vi "CAN_CANFD_Demo.vi"(11 "Receive":string="CAN_CANFD_Demo") -> ()   [LabVIEW 2014]
uses:
  <vilib>/Utility/miscctls.llb/LVPointTypeDef.ctl
  Utilities/Typedef/Hardware_Subtype.ctl
  TSMaster_API/CAN_CANFD_Function/Typedef/TSCAN_Config_parameter.ctl
  TSMaster_API/CAN_CANFD_Function/Typedef/TSCAN_Send_parameter.ctl
  TSMaster_API/CAN_CANFD_Function/Typedef/TSCAN_CAN_CANFD_Demo_Data.ctl
  TSMaster_API/CAN_CANFD_Function/Typedef/TSCAN_CAN_CANFD_Demo_Data1.ctl
  TSMaster_API/CAN_CANFD_Function/Typedef/TLibCANFD.ctl
  TSMaster_API/CAN_CANFD_Function/Typedef/TSCAN_DBC_Ctr.ctl
  TSMaster_API/CAN_CANFD_Function/Typedef/TSCAN_CANFD_Configuration.ctl
  TSMaster_API/CAN_CANFD_Function/Typedef/TSCAN_CAN_Configuration.ctl
  TSMaster_API/CAN_CANFD_Function/Typedef/TSCAN_CANFD_Configuration_Regs.ctl
  TSMaster_API/CAN_CANFD_Function/Typedef/TSCAN_CAN_Configuration_Regs.ctl
  TSMaster_API/All_Control/Typedef/Hardware Type.ctl
  TSMaster_API/All_Control/Typedef/Blf_Log.ctl
  TSMaster_API/DataBase/Typedef/DBSignal.ctl
  TSMaster_API/DataBase/Typedef/DBMessage.ctl
  <vilib>/regexp/Match Regular Expression.xnode
  TSMaster_API/Diagnosis/Typedef/UDS Control.ctl
  TSMaster_API/Diagnosis/Typedef/UDS Cluster.ctl
panel:
  in  "Diagram shown":bool
  in  "Stop Log":bool
  in  "Start Log":bool
  in  "log":i32(listbox)
  out "program loop":i32
  in  "Config":bool
  in  "Connect":bool
  in  "Disconnect":bool
  out "Connect ?":bool
  in  "选项卡控件":enum32{"Setting", "CAN/CANFD", "DBC_Load"}(tab)
  in  "CH_Mapping":bool
  in  "TS_Mapping":bool
  in  "BLF_Log_PATH":path
  in  "Advance_Tag":enum32{"Ordinary", "Advanced"}(tab)
  in  "CAN_Config_Array":T1[](array[typedef]) {"AAppChannel" items=["CHN1", "CHN2", "CHN3", "CHN4", "CHN5", "CHN6", "CHN7", "CHN8", "CHN9", "CHN10", "CHN11", "CHN12", "CHN13", "CHN14", "CHN15", "CHN16", "CHN17", "CHN18", "CHN19", "CHN20", "CHN21", "CHN22", "CHN23", "CHN24", "CHN25", "CHN26", "CHN27", "CHN28", "CHN29", "CHN30", "CHN31", "CHN32"]; "AHwChannel" items=["CHN1", "CHN2", "CHN3", "CHN4", "CHN5", "CHN6", "CHN7", "CHN8", "CHN9", "CHN10", "CHN11", "CHN12", "CHN13", "CHN14", "CHN15", "CHN16", "CHN17", "CHN18", "CHN19", "CHN20", "CHN21", "CHN22", "CHN23", "CHN24", "CHN25", "CHN26", "CHN27", "CHN28", "CHN29", "CHN30", "CHN31", "CHN32"]; "HardwareType" items=["BUS_UNKNOWN_TYPE", "TS_TCP_DEVICE", "XL_USB_DEVICE", "TS_USB_DEVICE", "PEAK_USB_DEVICE", "KVASER_USB_DEVICE", "ZLG_USB_DEVICE", "ICS_USB_DEVICE", "TS_TC1005_DEVICE", "CANABLE_USB_DEVICE", "TS_WIRELESS_OBD", "TS_USB_DEVICE_EX", "IXXAT_USB_DEVICE", "TS_ETH_IF_DEVICE", "TS_USB_IF_DEVICE", "BUS_DEV_TYPE_COUNT"]}
  in  "CANFD_Config_Array":T4[](array[typedef]) {"Hardware Type" items=["BUS_UNKNOWN_TYPE", "TS_TCP_DEVICE", "XL_USB_DEVICE", "TS_USB_DEVICE", "PEAK_USB_DEVICE", "KVASER_USB_DEVICE", "ZLG_USB_DEVICE", "ICS_USB_DEVICE", "TS_TC1005_DEVICE", "CANABLE_USB_DEVICE", "TS_WIRELESS_OBD", "TS_USB_DEVICE_EX", "IXXAT_USB_DEVICE", "TS_ETH_IF_DEVICE", "TS_USB_IF_DEVICE", "BUS_DEV_TYPE_COUNT"]; "AHwChannel" items=["CHN1", "CHN2", "CHN3", "CHN4", "CHN5", "CHN6", "CHN7", "CHN8", "CHN9", "CHN10", "CHN11", "CHN12", "CHN13", "CHN14", "CHN15", "CHN16", "CHN17", "CHN18", "CHN19", "CHN20", "CHN21", "CHN22", "CHN23", "CHN24", "CHN25", "CHN26", "CHN27", "CHN28", "CHN29", "CHN30", "CHN31", "CHN32"]; "AAppChannel" items=["CHN1", "CHN2", "CHN3", "CHN4", "CHN5", "CHN6", "CHN7", "CHN8", "CHN9", "CHN10", "CHN11", "CHN12", "CHN13", "CHN14", "CHN15", "CHN16", "CHN17", "CHN18", "CHN19", "CHN20", "CHN21", "CHN22", "CHN23", "CHN24", "CHN25", "CHN26", "CHN27", "CHN28", "CHN29", "CHN30", "CHN31", "CHN32"]; "AControllerType" items=["lfdtCAN", "lfdtISOFDCAN", "lfdtNonISOFDFDCAN"]; "AControllerMode" items=["lfdmNormal", "lfdmACKOff", "lfdmRestricted"]}
  in  "CANFD_Config_Regs_Array":T5[](array[typedef]) {"CANFD Configuration"."Hardware Type" items=["BUS_UNKNOWN_TYPE", "TS_TCP_DEVICE", "XL_USB_DEVICE", "TS_USB_DEVICE", "PEAK_USB_DEVICE", "KVASER_USB_DEVICE", "ZLG_USB_DEVICE", "ICS_USB_DEVICE", "TS_TC1005_DEVICE", "CANABLE_USB_DEVICE", "TS_WIRELESS_OBD", "TS_USB_DEVICE_EX", "IXXAT_USB_DEVICE", "TS_ETH_IF_DEVICE", "TS_USB_IF_DEVICE", "BUS_DEV_TYPE_COUNT"]; "CANFD Configuration"."AHwChannel" items=["CHN1", "CHN2", "CHN3", "CHN4", "CHN5", "CHN6", "CHN7", "CHN8", "CHN9", "CHN10", "CHN11", "CHN12", "CHN13", "CHN14", "CHN15", "CHN16", "CHN17", "CHN18", "CHN19", "CHN20", "CHN21", "CHN22", "CHN23", "CHN24", "CHN25", "CHN26", "CHN27", "CHN28", "CHN29", "CHN30", "CHN31", "CHN32"]; "CANFD Configuration"."AAppChannel" items=["CHN1", "CHN2", "CHN3", "CHN4", "CHN5", "CHN6", "CHN7", "CHN8", "CHN9", "CHN10", "CHN11", "CHN12", "CHN13", "CHN14", "CHN15", "CHN16", "CHN17", "CHN18", "CHN19", "CHN20", "CHN21", "CHN22", "CHN23", "CHN24", "CHN25", "CHN26", "CHN27", "CHN28", "CHN29", "CHN30", "CHN31", "CHN32"]; "CANFD Configuration"."AControllerType" items=["lfdtCAN", "lfdtISOFDCAN", "lfdtNonISOFDFDCAN"]; "CANFD Configuration"."AControllerMode" items=["lfdmNormal", "lfdmACKOff", "lfdmRestricted"]}
  in  "CAN_Config_Regs_Array":T6[](array[typedef]) {"CAN configuration"."AAppChannel" items=["CHN1", "CHN2", "CHN3", "CHN4", "CHN5", "CHN6", "CHN7", "CHN8", "CHN9", "CHN10", "CHN11", "CHN12", "CHN13", "CHN14", "CHN15", "CHN16", "CHN17", "CHN18", "CHN19", "CHN20", "CHN21", "CHN22", "CHN23", "CHN24", "CHN25", "CHN26", "CHN27", "CHN28", "CHN29", "CHN30", "CHN31", "CHN32"]; "CAN configuration"."AHwChannel" items=["CHN1", "CHN2", "CHN3", "CHN4", "CHN5", "CHN6", "CHN7", "CHN8", "CHN9", "CHN10", "CHN11", "CHN12", "CHN13", "CHN14", "CHN15", "CHN16", "CHN17", "CHN18", "CHN19", "CHN20", "CHN21", "CHN22", "CHN23", "CHN24", "CHN25", "CHN26", "CHN27", "CHN28", "CHN29", "CHN30", "CHN31", "CHN32"]; "CAN configuration"."HardwareType" items=["BUS_UNKNOWN_TYPE", "TS_TCP_DEVICE", "XL_USB_DEVICE", "TS_USB_DEVICE", "PEAK_USB_DEVICE", "KVASER_USB_DEVICE", "ZLG_USB_DEVICE", "ICS_USB_DEVICE", "TS_TC1005_DEVICE", "CANABLE_USB_DEVICE", "TS_WIRELESS_OBD", "TS_USB_DEVICE_EX", "IXXAT_USB_DEVICE", "TS_ETH_IF_DEVICE", "TS_USB_IF_DEVICE", "BUS_DEV_TYPE_COUNT"]}
  in  "DLL_PATH":path
  in  "Bus_Type":u16(ring) items=["CAN", "CANFD"]
  in  "Channels used":u16(ring)=1 items=["1 Channel"=1, "2 Channels"=2, "3 Channels"=3, "4 Channels"=4, "5 Channels"=5, "6 Channels"=6, "7 Channels"=7, "8 Channels"=8, "9 Channels"=9, "10 Channels"=10, "11 Channels"=11, "12 Channels"=12, "13 Channels"=13, "14 Channels"=14, "15 Channels"=15, "16 Channels"=16]
  in  "Sampling point":bool
  in  "Export":bool
  in  "Import":bool
  in  "REC_Channel":i32(ring) items=["CHN1", "CHN2", "CHN3", "CHN4", "CHN5", "CHN6", "CHN7", "CHN8", "CHN9", "CHN10", "CHN11", "CHN12", "CHN13", "CHN14", "CHN15", "CHN16", "CHN17", "CHN18", "CHN19", "CHN20", "CHN21", "CHN22", "CHN23", "CHN24", "CHN25", "CHN26", "CHN27", "CHN28", "CHN29", "CHN30", "CHN31", "CHN32"]
  in  "DIS_REC":bool
  in  "Pause":bool
  in  "Read message type":u16(ring)=1 items=["Only read received messages", "Receive&send messages"]
  out "Receive Status":bool
  in  "Clear":bool
  in  "BRS":enum16{"Close", "Open"}(ring)
  in  "FD Frame":u8(ring) items=["Ordinary CAN Data", "FD CAN Data"]
  in  "Frame Type":u8(ring) items=["Data Frame", "Remote Frame", ""]
  in  "Frame Format":u8(ring) items=["Standard Frame", "Extended Frame"]
  in  "ID":i32 format="%x"
  in  "Data Length":i32(ring)=15 items=["0", "1", "2", "3", "4", "5", "6", "7", "8", "12", "16", "20", "24", "32", "48", "64"]
  in  "SendData":u8[](array[numeric])=[0, 0, 0, 0, 0, 0, 0, 0, 0, 0, 0, 0, 0, 0, 0, 0, 0, 0, 0, 0, 0, 0, 0, 0, 0, 0, 0, 0, 0, 0, 0, 0, 0, 0, 0, 0, 0, 0, 0, 0, 0, 0, 0, 0, 0, 0, 0, 0, 0, 0, 0, 0, 0, 0, 0, 0, 0, 0, 0, 0, 0, 0, 0, 0, 0, 0, 0, 0, 0, 0, 0, 0, 0, 0, 0] format="%x"
  in  "Data":i32(listbox)=-1
  in  "Send_Tag":T7(tab)
  out "ms":u32
  out "send successful?":bool
  in  "Sending":bool
  in  "Cycle":bool=TRUE
  in  "Channel":i32(ring) items=["CHN1", "CHN2", "CHN3", "CHN4", "CHN5", "CHN6", "CHN7", "CHN8", "CHN9", "CHN10", "CHN11", "CHN12", "CHN13", "CHN14", "CHN15", "CHN16", "CHN17", "CHN18", "CHN19", "CHN20", "CHN21", "CHN22", "CHN23", "CHN24", "CHN25", "CHN26", "CHN27", "CHN28", "CHN29", "CHN30", "CHN31", "CHN32"]
  in  "async&sync":u16(ring) items=["async", "sync"]
  in  "Timeout":u16
  in  "Periodic_Send":bool
  in  "Filtering":bool
  in  "DBC_Send":bool
  in  "AsynCall":bool
  in  "UDS":bool
  out "BufferCount":i32
  out "ok?":bool
  out "State":dbl
  out "Stste?":bool
  in  "AIdxStat":i32(ring) items=["cbsBusLoad", "cbsPeakLoad", "cbsFpsStdData", "cbsAllStdData", "cbsFpsExtData", "cbsAllExtData", "cbsFpsStdRemote", "cbsAllStdRemote", "cbsFpsExtRemote", "cbsAllExtRemote", "cbsFpsErrorFrame", "cbsAllErrorFrame"]
  in  "Fold Data":bool
  out "Laod BDC Successful?":bool
  in  "DBC Tab":enum32{"Message", "Signal"}(tab) caption="Tab Control 2"
  in  "Message Table":string[][](table)=[["Name", ""], ["Type", ""], ["Data Length", ""], ["Identifier", ""], ["Baud rate switching flag", ""], ["Cycle (milliseconds)", ""], ["Annotation", ""]]
  in  "Signal Table":string[][](table)=[["Name", ""], ["Length", ""], ["Endian", ""], ["DataType", ""], ["Minimum", ""], ["Maximum", ""], ["Unit", ""], ["Factor", ""], ["Offset", ""], ["InitiaValue", ""], ["Annotation", ""]]
  in  "GetCount_DBC":bool
  in  "Unload_DBC":bool
  in  "Load_DBC":bool
  in  "Tree control":string(tree)
  in  "DBC loading channel":i32(ring) items=["CHN1", "CHN2", "CHN3", "CHN4", "CHN5", "CHN6", "CHN7", "CHN8", "CHN9", "CHN10", "CHN11", "CHN12", "CHN13", "CHN14", "CHN15", "CHN16", "CHN17", "CHN18", "CHN19", "CHN20", "CHN21", "CHN22", "CHN23", "CHN24", "CHN25", "CHN26", "CHN27", "CHN28", "CHN29", "CHN30", "CHN31", "CHN32"]
  in  "DBC Path":path
  in  "STOP":bool
  # "CAN/CANFD Demo"
  # "Please click the 'Config' button first,Don't click \"Connect\""
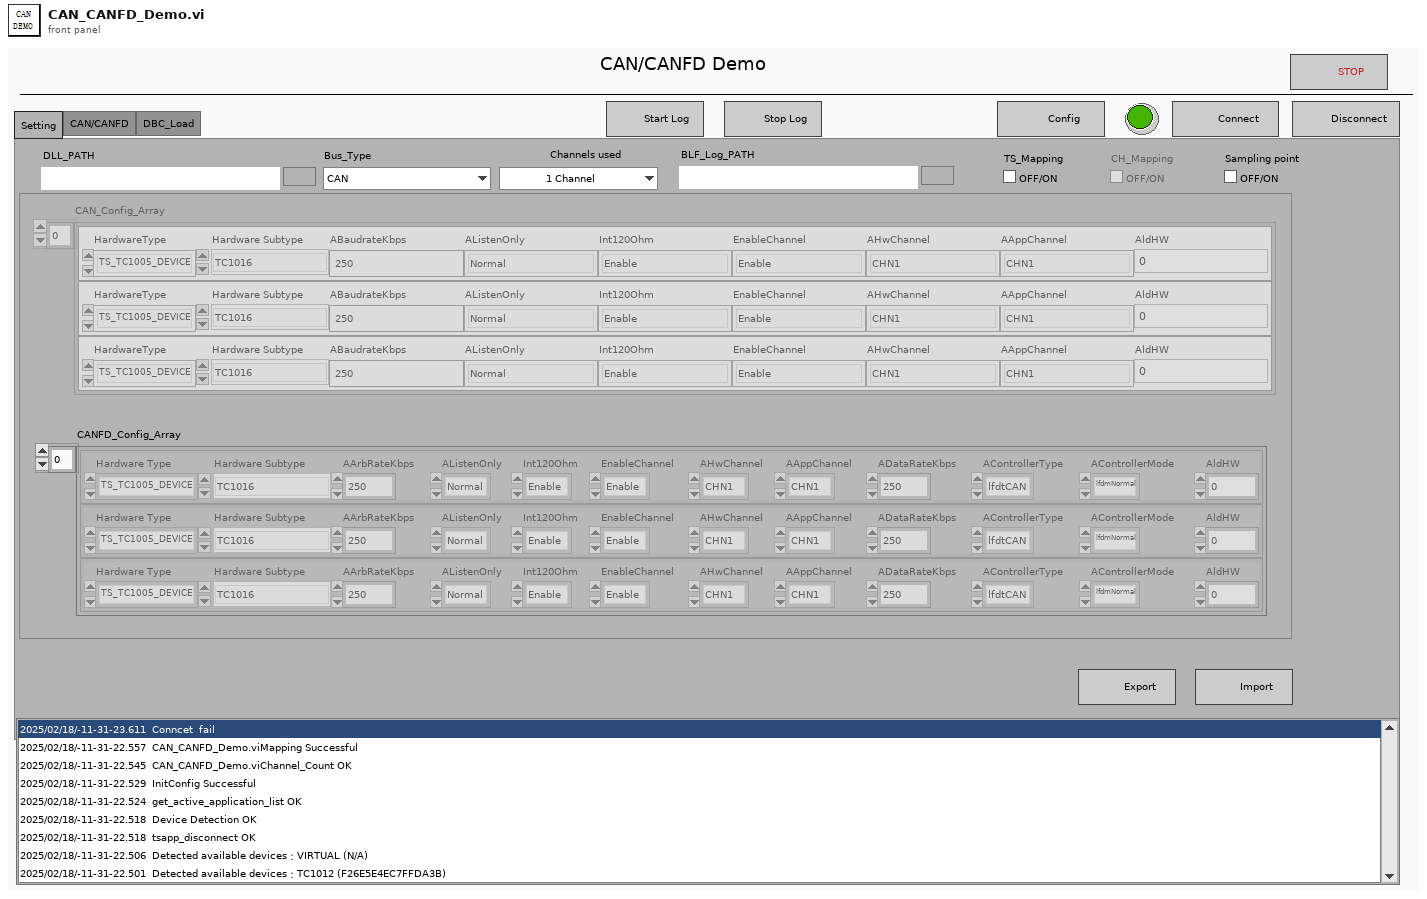
[diagram p1: front panel]
types:
  T1 = typedef "TSCAN_CAN_Configuration.ctl" = cluster{"HardwareType":T2, "Hardware Subtype":T3, "ABaudrateKbps":sgl, "AListenOnly":enum16{"Normal", "ListenOnly"}, "Int120Ohm":enum16{"Disable", "Enable"}, "EnableChannel":enum16{"Disable", "Enable"}, "AHwChannel":i32, "AAppChannel":i32, "AldHW":i32}
  T2 = typedef "Hardware Type.ctl" = i32
  T3 = typedef "Hardware_Subtype.ctl" = enum16{"TS_UNKNOWN_DEVICE", "TSCAN_PRO", "TSCAN_Lite1", "TC1001", "TL1001", "TC1011", "TM5011", "TC1002", "TC1014", "TSCANFD2517", "TC1026", "TC1016", "TC1012", "TC1013", "TLog1002", "TC1034", "TC1018", "GW2116", "TC2115", "MP1013", "TC1113", "TC1114", "TP1013", "TC1017", "TP1018", "TF10XX", "TL1004_FD_4_LIN_2", "TE1051", "TP1051", "TP1034", "TTS9015", "TP1026", "TTS1026", "TTS1034", "TTS1018", "TL1011", "TTS1015_LiAuto", "TTS1013_LiAuto", "TTS1016Pro", "TC1054Pro", "TC1054", "TLog1038", "TO1013", "TC1034Pro", "TC1018Pro", "TC1038Pro", "TS_DEV_END"}
  T4 = typedef "TSCAN_CANFD_Configuration.ctl" = cluster{"Hardware Type":T2, "Hardware Subtype":T3, "AArbRateKbps":sgl, "AListenOnly":enum16{"Normal", "ListenOnly"}, "Int120Ohm":enum16{"Disable", "Enable"}, "EnableChannel":enum16{"Disable", "Enable"}, "AHwChannel":i32, "AAppChannel":i32, "ADataRateKbps":sgl, "AControllerType":i32, "AControllerMode":i32, "AldHW":i32}
  T5 = typedef "TSCAN_CANFD_Configuration_Regs.ctl" = cluster{"CANFD Configuration":T4, "CANFD_Sampling point":cluster{"AArbSEG1":i32, "AArbSEG2":i32, "AArbPrescaler":i32, "AArbSJW":i32, "ADataSEG1":i32, "ADataSEG2":i32, "ADataPrescaler":i32, "ADataSJW":i32}}
  T6 = typedef "TSCAN_CAN_Configuration_Regs.ctl" = cluster{"CAN_Sampling point":cluster{"ASEG1":i32, "ASEG2":i32, "APrescaler":i32, "ASJW":i32}, "CAN configuration":T1}
  T7 = enum32{"Single step", "Periodic", "Filter_Pass", "DBC", "UDS"}
  T8 = enum8{"Enabled", "Disabled", "Disabled and Grayed Out"}
  T9 = typedef "LVPointTypeDef.ctl" = cluster{"Horizontal":i16, "Vertical":i16}
  T10 = typedef "TSCAN_CAN_CANFD_Demo_Data1.ctl" = cluster{"Communication message":cluster{"Sender":string, "receiver":string, "message":string, "data":variant}, "Data":T11, "CAN_Buffer":cluster{"FIdxChn":u8, "FProperties":u8, "FDLC":u8, "FReserved":u8, "FIdentifier":i32, "FTimeUS":u64, "FData":cluster{"Data0":u8, "Data1":u8, "Data2":u8, "Data3":u8, "Data4":u8, "Data5":u8, "Data6":u8, "Data7":u8}}[], "CANFD_Buffer":cluster{"FIdxChn":u8, "FProperties":u8, "FDLC":u8, "FReserved":u8, "FIdentifier":i32, "FTimeUS":u64, "FDatas":cluster{"Initialize array[0]":u8, "Initialize array[1]":u8, "Initialize array[2]":u8, "Initialize array[3]":u8, "Initialize array[4]":u8, "Initialize array[5]":u8, "Initialize array[6]":u8, "Initialize array[7]":u8, "Initialize array[8]":u8, "Initialize array[9]":u8, "Initialize array[10]":u8, "Initialize array[11]":u8, "Initialize array[12]":u8, "Initialize array[13]":u8, "Initialize array[14]":u8, "Initialize array[15]":u8, "Initialize array[16]":u8, "Initialize array[17]":u8, "Initialize array[18]":u8, "Initialize array[19]":u8, "Initialize array[20]":u8, "Initialize array[21]":u8, "Initialize array[22]":u8, "Initialize array[23]":u8, "Initialize array[24]":u8, "Initialize array[25]":u8, "Initialize array[26]":u8, "Initialize array[27]":u8, "Initialize array[28]":u8, "Initialize array[29]":u8, "Initialize array[30]":u8, "Initialize array[31]":u8, "Initialize array[32]":u8, "Initialize array[33]":u8, "Initialize array[34]":u8, "Initialize array[35]":u8, "Initialize array[36]":u8, "Initialize array[37]":u8, "Initialize array[38]":u8, "Initialize array[39]":u8, "Initialize array[40]":u8, "Initialize array[41]":u8, "Initialize array[42]":u8, "Initialize array[43]":u8, "Initialize array[44]":u8, "Initialize array[45]":u8, "Initialize array[46]":u8, "Initialize array[47]":u8, "Initialize array[48]":u8, "Initialize array[49]":u8, "Initialize array[50]":u8, "Initialize array[51]":u8, "Initialize array[52]":u8, "Initialize array[53]":u8, "Initialize array[54]":u8, "Initialize array[55]":u8, "Initialize array[56]":u8, "Initialize array[57]":u8, "Initialize array[58]":u8, "Initialize array[59]":u8, "Initialize array[60]":u8, "Initialize array[61]":u8, "Initialize array[62]":u8, "Initialize array[63]":u8}}[], "error in":errorcluster, "CAN_Period_Datas":cluster{"FIdxChn":u8, "FProperties":u8, "FDLC":u8, "FReserved":u8, "FIdentifier":i32, "FTimeUS":u64, "FData":cluster{"Data0":u8, "Data1":u8, "Data2":u8, "Data3":u8, "Data4":u8, "Data5":u8, "Data6":u8, "Data7":u8}}[], "CANFD_period_Datas":cluster{"FIdxChn":u8, "FProperties":u8, "FDLC":u8, "FReserved":u8, "FIdentifier":i32, "FTimeUS":u64, "FDatas":cluster{"Initialize array[0]":u8, "Initialize array[1]":u8, "Initialize array[2]":u8, "Initialize array[3]":u8, "Initialize array[4]":u8, "Initialize array[5]":u8, "Initialize array[6]":u8, "Initialize array[7]":u8, "Initialize array[8]":u8, "Initialize array[9]":u8, "Initialize array[10]":u8, "Initialize array[11]":u8, "Initialize array[12]":u8, "Initialize array[13]":u8, "Initialize array[14]":u8, "Initialize array[15]":u8, "Initialize array[16]":u8, "Initialize array[17]":u8, "Initialize array[18]":u8, "Initialize array[19]":u8, "Initialize array[20]":u8, "Initialize array[21]":u8, "Initialize array[22]":u8, "Initialize array[23]":u8, "Initialize array[24]":u8, "Initialize array[25]":u8, "Initialize array[26]":u8, "Initialize array[27]":u8, "Initialize array[28]":u8, "Initialize array[29]":u8, "Initialize array[30]":u8, "Initialize array[31]":u8, "Initialize array[32]":u8, "Initialize array[33]":u8, "Initialize array[34]":u8, "Initialize array[35]":u8, "Initialize array[36]":u8, "Initialize array[37]":u8, "Initialize array[38]":u8, "Initialize array[39]":u8, "Initialize array[40]":u8, "Initialize array[41]":u8, "Initialize array[42]":u8, "Initialize array[43]":u8, "Initialize array[44]":u8, "Initialize array[45]":u8, "Initialize array[46]":u8, "Initialize array[47]":u8, "Initialize array[48]":u8, "Initialize array[49]":u8, "Initialize array[50]":u8, "Initialize array[51]":u8, "Initialize array[52]":u8, "Initialize array[53]":u8, "Initialize array[54]":u8, "Initialize array[55]":u8, "Initialize array[56]":u8, "Initialize array[57]":u8, "Initialize array[58]":u8, "Initialize array[59]":u8, "Initialize array[60]":u8, "Initialize array[61]":u8, "Initialize array[62]":u8, "Initialize array[63]":u8}}[], "CAN_Filtering_Datas":cluster{"FIdxChn":u8, "FProperties":u8, "FDLC":u8, "FReserved":u8, "FIdentifier":i32, "FTimeUS":u64, "FData":cluster{"Data0":u8, "Data1":u8, "Data2":u8, "Data3":u8, "Data4":u8, "Data5":u8, "Data6":u8, "Data7":u8}}[], "CANFD_Filtering_Datas":cluster{"FIdxChn":u8, "FProperties":u8, "FDLC":u8, "FReserved":u8, "FIdentifier":i32, "FTimeUS":u64, "FDatas":cluster{"Initialize array[0]":u8, "Initialize array[1]":u8, "Initialize array[2]":u8, "Initialize array[3]":u8, "Initialize array[4]":u8, "Initialize array[5]":u8, "Initialize array[6]":u8, "Initialize array[7]":u8, "Initialize array[8]":u8, "Initialize array[9]":u8, "Initialize array[10]":u8, "Initialize array[11]":u8, "Initialize array[12]":u8, "Initialize array[13]":u8, "Initialize array[14]":u8, "Initialize array[15]":u8, "Initialize array[16]":u8, "Initialize array[17]":u8, "Initialize array[18]":u8, "Initialize array[19]":u8, "Initialize array[20]":u8, "Initialize array[21]":u8, "Initialize array[22]":u8, "Initialize array[23]":u8, "Initialize array[24]":u8, "Initialize array[25]":u8, "Initialize array[26]":u8, "Initialize array[27]":u8, "Initialize array[28]":u8, "Initialize array[29]":u8, "Initialize array[30]":u8, "Initialize array[31]":u8, "Initialize array[32]":u8, "Initialize array[33]":u8, "Initialize array[34]":u8, "Initialize array[35]":u8, "Initialize array[36]":u8, "Initialize array[37]":u8, "Initialize array[38]":u8, "Initialize array[39]":u8, "Initialize array[40]":u8, "Initialize array[41]":u8, "Initialize array[42]":u8, "Initialize array[43]":u8, "Initialize array[44]":u8, "Initialize array[45]":u8, "Initialize array[46]":u8, "Initialize array[47]":u8, "Initialize array[48]":u8, "Initialize array[49]":u8, "Initialize array[50]":u8, "Initialize array[51]":u8, "Initialize array[52]":u8, "Initialize array[53]":u8, "Initialize array[54]":u8, "Initialize array[55]":u8, "Initialize array[56]":u8, "Initialize array[57]":u8, "Initialize array[58]":u8, "Initialize array[59]":u8, "Initialize array[60]":u8, "Initialize array[61]":u8, "Initialize array[62]":u8, "Initialize array[63]":u8}}[], "AsynCall?":bool}
  T11 = typedef "TSCAN_CAN_CANFD_Demo_Data.ctl" = cluster{"Config_parameter":T12, "Send_parameter":T13, "DBC_Ctr":T14, "CAN_Config_Array":T1[], "CANFD_Config_Array":T4[], "CAN_Config_Regs_Array":T6[], "CANFD_Config_Regs_Array":T5[], "Blf_Log":T17, "UDS":T18}
  T12 = typedef "TSCAN_Config_parameter.ctl" = cluster{"Bus_Type":u16, "Channel":i32, "Channels used":u16, "DLL_PATH":path, "Read message type":u16, "REC_Channel":i32}
  T13 = typedef "TSCAN_Send_parameter.ctl" = cluster{"SendData":u8[], "Data Length":i32, "ID":i32, "Frame Format":u8, "Frame Type":u8, "BRS":enum16{"Close", "Open"}, "FD Frame":u8, "async&sync":enum16{"async", "sync"}, "Timeout":u16}
  T14 = typedef "TSCAN_DBC_Ctr.ctl" = cluster{"DBC Path":path, "DBC loading channel":i32, "DatabaseId":u32, "DBMessages":T15[], "DBSignals":cluster{"MessageName":string, "SignalList":T16[]}[]}
  T15 = typedef "DBMessage.ctl" = cluster{"Type":u16, "DLC":i32, "ID":i32, "CycleTime":dbl, "Name":string, "Comment":string, "TX_Node_Index":i32, "Owned_Signal_List_Count ":i32, "Owned_Signal_List_Signal_Index":i32, "BRS":i32}
  T16 = typedef "DBSignal.ctl" = cluster{"ID":i32, "Value_Type":i32, "Is_Motorola":i32, "ValTab_Index":i32, "Mux_Type":i32, "Mux_Value":dbl, "Layout_Start":i32, "Length":i32, "Factor":dbl, "Offset":dbl, "InitValue":dbl, "Min":dbl, "Max":dbl, "Name":string, "Unit":string, "Comment":string, "Message_Index":i32, "Message_Type":i32}
  T17 = typedef "Blf_Log.ctl" = cluster{"Blf_Log_PATH":path}
  T18 = typedef "UDS Cluster.ctl" = cluster{"UDS Control":T19, "DiagModuleIndex":i32}
  T19 = typedef "UDS Control.ctl" = cluster{"UDS Channel Index":u32, "Request ID":u32, "Response ID":u32, "Request ID (Func)":u32, "Session Mode":u8, "Reset Mode":u8, "DTC Mask":u8, "GropOfDTC":u32, "Seed Level":i32, "Seed":u8[], "Key Level":i32, "Key":u8[], "Read Identifier":u16, "UDS Read Data":u8[], "ASCII Data":string, "Write Identifier":u16, "UDS Wrtie Data":u8[], "IO Control Identifier":u16, "UDS IOControl Data":u8[], "IO Control Mode":u8, "UDS IOControl Read Data":u8[], "Routine Control Identifier":u16, "UDS RoutineControl Data":u8[], "UDS RoutineControl Read Data":u8[], "Routine Control Mode":u8, "SupportFDCAN":bool, "time config":cluster{"p2_timeout":i32, "p2_extended":i32, "s3_servertime":i32, "s3_clienttime":i32}, "ServiceLayer":cluster{"FilledByte":u8, "STMin":i32, "BlockSize":i32, "FCDelay":i32, "MaxLength":i32}, "Request":u8[], "Respond":u8[]}
  T20 = cluster{"Sender":string, "receiver":string, "message":string, "data":variant}
  T21 = cluster{"FIdxChn":u8, "FProperties":u8, "FDLC":u8, "FReserved":u8, "FIdentifier":i32, "FTimeUS":u64, "FData":cluster{"Data0":u8, "Data1":u8, "Data2":u8, "Data3":u8, "Data4":u8, "Data5":u8, "Data6":u8, "Data7":u8}}[]
  T22 = cluster{"FIdxChn":u8, "FProperties":u8, "FDLC":u8, "FReserved":u8, "FIdentifier":i32, "FTimeUS":u64, "FDatas":cluster{"Initialize array[0]":u8, "Initialize array[1]":u8, "Initialize array[2]":u8, "Initialize array[3]":u8, "Initialize array[4]":u8, "Initialize array[5]":u8, "Initialize array[6]":u8, "Initialize array[7]":u8, "Initialize array[8]":u8, "Initialize array[9]":u8, "Initialize array[10]":u8, "Initialize array[11]":u8, "Initialize array[12]":u8, "Initialize array[13]":u8, "Initialize array[14]":u8, "Initialize array[15]":u8, "Initialize array[16]":u8, "Initialize array[17]":u8, "Initialize array[18]":u8, "Initialize array[19]":u8, "Initialize array[20]":u8, "Initialize array[21]":u8, "Initialize array[22]":u8, "Initialize array[23]":u8, "Initialize array[24]":u8, "Initialize array[25]":u8, "Initialize array[26]":u8, "Initialize array[27]":u8, "Initialize array[28]":u8, "Initialize array[29]":u8, "Initialize array[30]":u8, "Initialize array[31]":u8, "Initialize array[32]":u8, "Initialize array[33]":u8, "Initialize array[34]":u8, "Initialize array[35]":u8, "Initialize array[36]":u8, "Initialize array[37]":u8, "Initialize array[38]":u8, "Initialize array[39]":u8, "Initialize array[40]":u8, "Initialize array[41]":u8, "Initialize array[42]":u8, "Initialize array[43]":u8, "Initialize array[44]":u8, "Initialize array[45]":u8, "Initialize array[46]":u8, "Initialize array[47]":u8, "Initialize array[48]":u8, "Initialize array[49]":u8, "Initialize array[50]":u8, "Initialize array[51]":u8, "Initialize array[52]":u8, "Initialize array[53]":u8, "Initialize array[54]":u8, "Initialize array[55]":u8, "Initialize array[56]":u8, "Initialize array[57]":u8, "Initialize array[58]":u8, "Initialize array[59]":u8, "Initialize array[60]":u8, "Initialize array[61]":u8, "Initialize array[62]":u8, "Initialize array[63]":u8}}[]
  T23 = cluster{"Channel select":u8, "ID":i32, "Frame format":u8, "Frame type":u8, "Length":u8, "Data":cluster{"Data0":u8, "Data1":u8, "Data2":u8, "Data3":u8, "Data4":u8, "Data5":u8, "Data6":u8, "Data7":u8}}
  T24 = typedef "TLibCANFD.ctl" = cluster{"AIdxchn":u8, "AId":i32, "AIsStd":u8, "BRS":enum16{"Close", "Open"}, "AIsData":u8, "ADLC":i32, "AIsFD":enum16{"Classic CAN Message", "FD CAN Message"}, "FDatas":cluster{"Initialize array[0]":u8, "Initialize array[1]":u8, "Initialize array[2]":u8, "Initialize array[3]":u8, "Initialize array[4]":u8, "Initialize array[5]":u8, "Initialize array[6]":u8, "Initialize array[7]":u8, "Initialize array[8]":u8, "Initialize array[9]":u8, "Initialize array[10]":u8, "Initialize array[11]":u8, "Initialize array[12]":u8, "Initialize array[13]":u8, "Initialize array[14]":u8, "Initialize array[15]":u8, "Initialize array[16]":u8, "Initialize array[17]":u8, "Initialize array[18]":u8, "Initialize array[19]":u8, "Initialize array[20]":u8, "Initialize array[21]":u8, "Initialize array[22]":u8, "Initialize array[23]":u8, "Initialize array[24]":u8, "Initialize array[25]":u8, "Initialize array[26]":u8, "Initialize array[27]":u8, "Initialize array[28]":u8, "Initialize array[29]":u8, "Initialize array[30]":u8, "Initialize array[31]":u8, "Initialize array[32]":u8, "Initialize array[33]":u8, "Initialize array[34]":u8, "Initialize array[35]":u8, "Initialize array[36]":u8, "Initialize array[37]":u8, "Initialize array[38]":u8, "Initialize array[39]":u8, "Initialize array[40]":u8, "Initialize array[41]":u8, "Initialize array[42]":u8, "Initialize array[43]":u8, "Initialize array[44]":u8, "Initialize array[45]":u8, "Initialize array[46]":u8, "Initialize array[47]":u8, "Initialize array[48]":u8, "Initialize array[49]":u8, "Initialize array[50]":u8, "Initialize array[51]":u8, "Initialize array[52]":u8, "Initialize array[53]":u8, "Initialize array[54]":u8, "Initialize array[55]":u8, "Initialize array[56]":u8, "Initialize array[57]":u8, "Initialize array[58]":u8, "Initialize array[59]":u8, "Initialize array[60]":u8, "Initialize array[61]":u8, "Initialize array[62]":u8, "Initialize array[63]":u8}}
  T25 = cluster{"MessageName":string, "SignalList":T16[]}[]
  T26 = cluster{"FIdxChn":u8, "FProperties":u8, "FDLC":u8, "FReserved":u8, "FIdentifier":i32, "FTimeUS":u64, "Fdata":cluster{"初始化的数组[0]":u8, "初始化的数组[1]":u8, "初始化的数组[2]":u8, "初始化的数组[3]":u8, "初始化的数组[4]":u8, "初始化的数组[5]":u8, "初始化的数组[6]":u8, "初始化的数组[7]":u8, "初始化的数组[8]":u8, "初始化的数组[9]":u8, "初始化的数组[10]":u8, "初始化的数组[11]":u8, "初始化的数组[12]":u8, "初始化的数组[13]":u8, "初始化的数组[14]":u8, "初始化的数组[15]":u8, "初始化的数组[16]":u8, "初始化的数组[17]":u8, "初始化的数组[18]":u8, "初始化的数组[19]":u8, "初始化的数组[20]":u8, "初始化的数组[21]":u8, "初始化的数组[22]":u8, "初始化的数组[23]":u8, "初始化的数组[24]":u8, "初始化的数组[25]":u8, "初始化的数组[26]":u8, "初始化的数组[27]":u8, "初始化的数组[28]":u8, "初始化的数组[29]":u8, "初始化的数组[30]":u8, "初始化的数组[31]":u8, "初始化的数组[32]":u8, "初始化的数组[33]":u8, "初始化的数组[34]":u8, "初始化的数组[35]":u8, "初始化的数组[36]":u8, "初始化的数组[37]":u8, "初始化的数组[38]":u8, "初始化的数组[39]":u8, "初始化的数组[40]":u8, "初始化的数组[41]":u8, "初始化的数组[42]":u8, "初始化的数组[43]":u8, "初始化的数组[44]":u8, "初始化的数组[45]":u8, "初始化的数组[46]":u8, "初始化的数组[47]":u8, "初始化的数组[48]":u8, "初始化的数组[49]":u8, "初始化的数组[50]":u8, "初始化的数组[51]":u8, "初始化的数组[52]":u8, "初始化的数组[53]":u8, "初始化的数组[54]":u8, "初始化的数组[55]":u8, "初始化的数组[56]":u8, "初始化的数组[57]":u8, "初始化的数组[58]":u8, "初始化的数组[59]":u8, "初始化的数组[60]":u8, "初始化的数组[61]":u8, "初始化的数组[62]":u8, "初始化的数组[63]":u8}}[]
  T27 = cluster{"SendData[0]":u8, "SendData[1]":u8, "SendData[2]":u8, "SendData[3]":u8, "SendData[4]":u8, "SendData[5]":u8, "SendData[6]":u8, "SendData[7]":u8}
  T28 = cluster{"SendData[0]":u8, "SendData[1]":u8, "SendData[2]":u8, "SendData[3]":u8, "SendData[4]":u8, "SendData[5]":u8, "SendData[6]":u8, "SendData[7]":u8, "SendData[8]":u8, "SendData[9]":u8, "SendData[10]":u8, "SendData[11]":u8, "SendData[12]":u8, "SendData[13]":u8, "SendData[14]":u8, "SendData[15]":u8, "SendData[16]":u8, "SendData[17]":u8, "SendData[18]":u8, "SendData[19]":u8, "SendData[20]":u8, "SendData[21]":u8, "SendData[22]":u8, "SendData[23]":u8, "SendData[24]":u8, "SendData[25]":u8, "SendData[26]":u8, "SendData[27]":u8, "SendData[28]":u8, "SendData[29]":u8, "SendData[30]":u8, "SendData[31]":u8, "SendData[32]":u8, "SendData[33]":u8, "SendData[34]":u8, "SendData[35]":u8, "SendData[36]":u8, "SendData[37]":u8, "SendData[38]":u8, "SendData[39]":u8, "SendData[40]":u8, "SendData[41]":u8, "SendData[42]":u8, "SendData[43]":u8, "SendData[44]":u8, "SendData[45]":u8, "SendData[46]":u8, "SendData[47]":u8, "SendData[48]":u8, "SendData[49]":u8, "SendData[50]":u8, "SendData[51]":u8, "SendData[52]":u8, "SendData[53]":u8, "SendData[54]":u8, "SendData[55]":u8, "SendData[56]":u8, "SendData[57]":u8, "SendData[58]":u8, "SendData[59]":u8, "SendData[60]":u8, "SendData[61]":u8, "SendData[62]":u8, "SendData[63]":u8}
  T29 = cluster{"Node_Name":string, "Node_Addres":i32, "Node_Commet":string, "Node_TX_List":cluster{"Name":string, "ID":i32}[], "Node_RX_List":cluster{"Name":string, "ID":i32}[]}[]
  T30 = enum32{"invalid app kind", "Development System", "Run Time System", "Student Edition", "Embedded LabVIEW", "Evaluation", "Custom"}
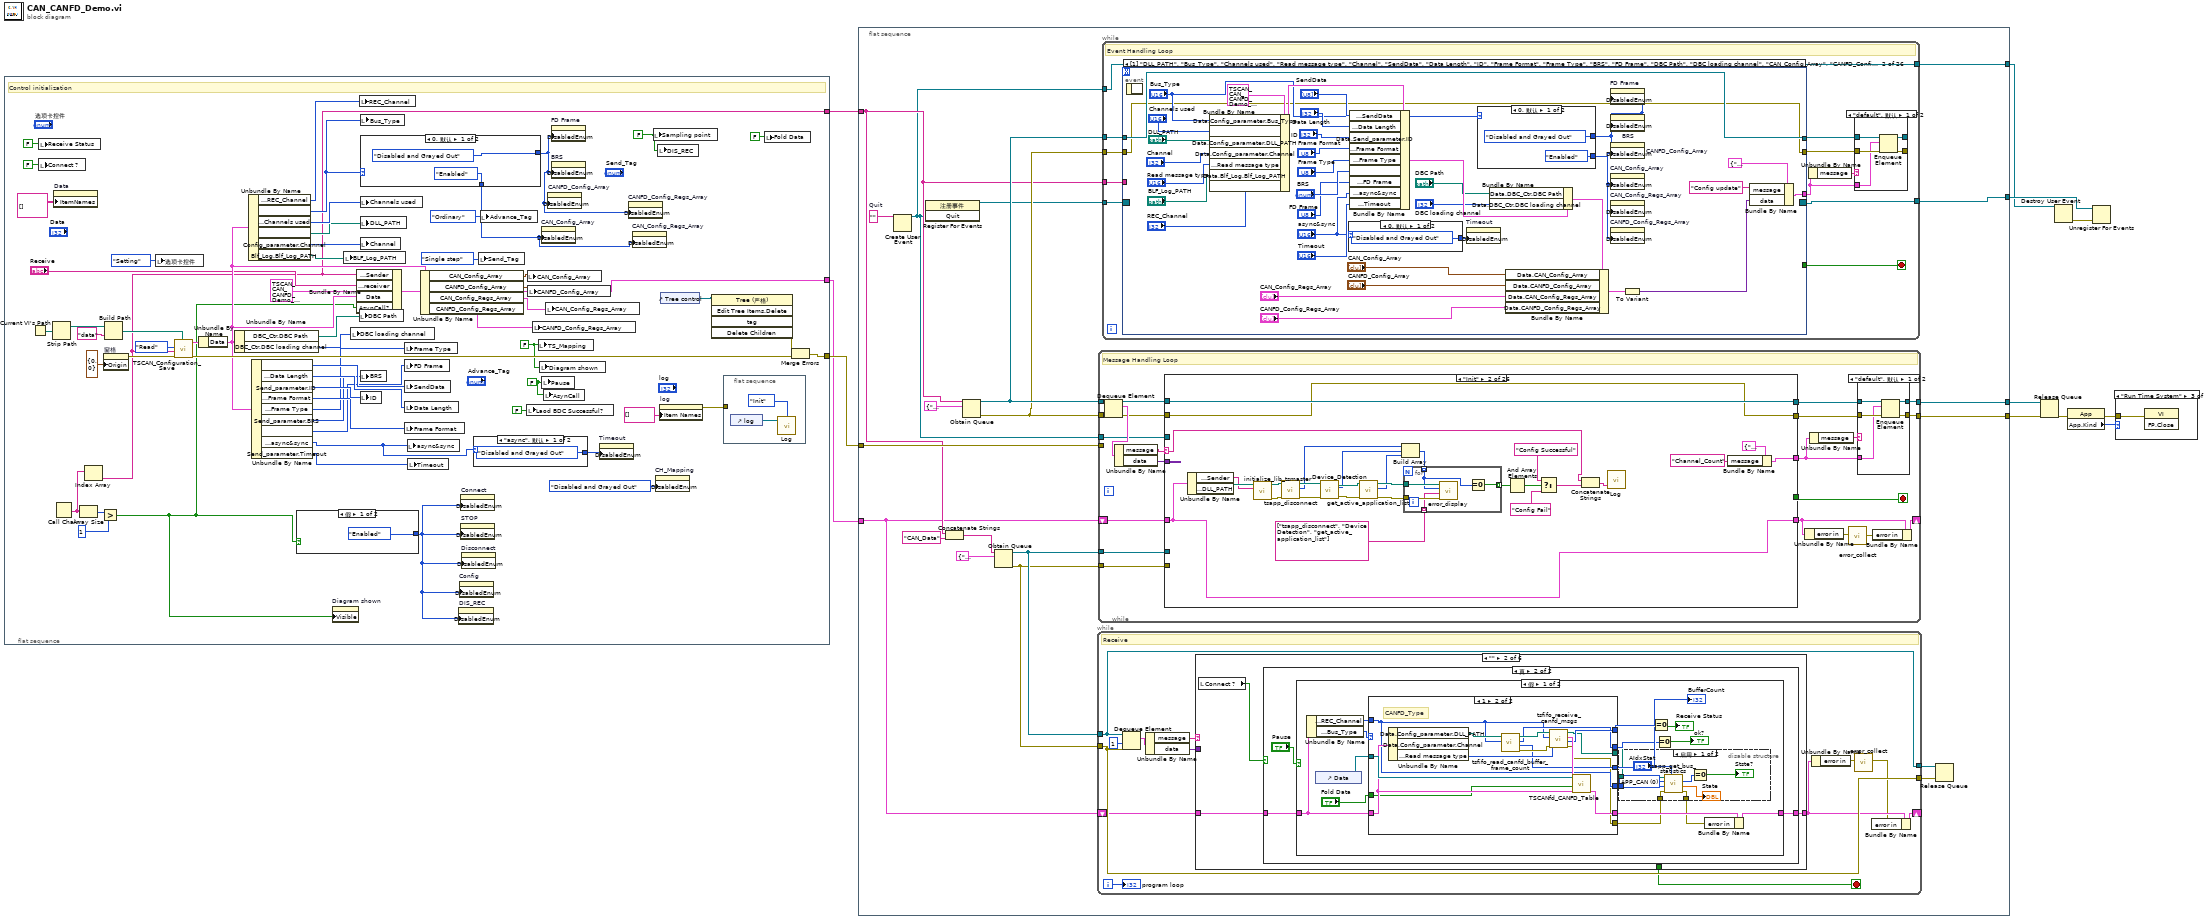
[diagram p0: block diagram]
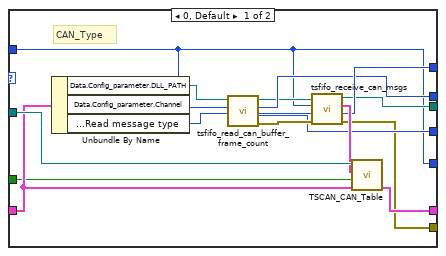
[diagram p5: hidden frame]
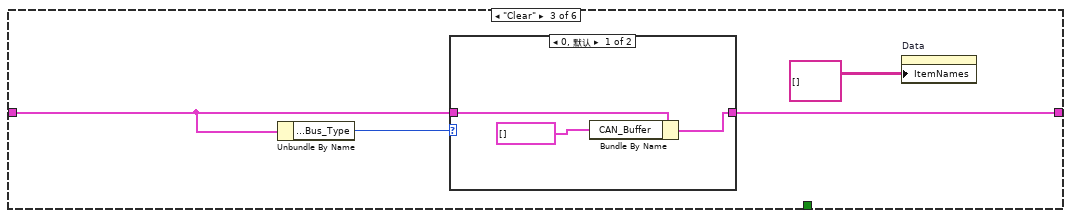
[diagram p7: hidden frame]
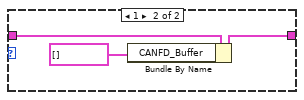
[diagram p8: hidden frame]
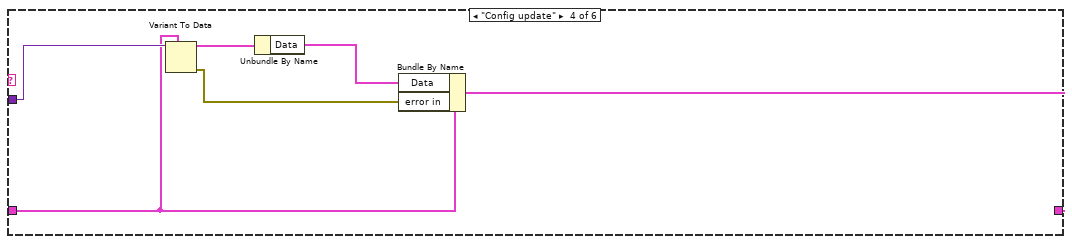
[diagram p9: hidden frame]
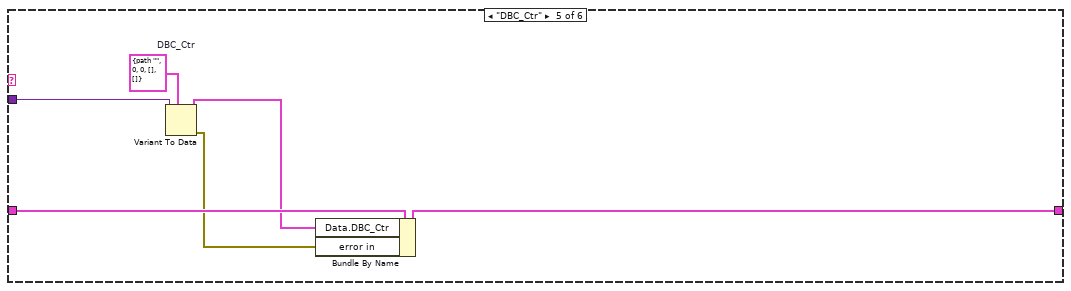
[diagram p10: hidden frame]
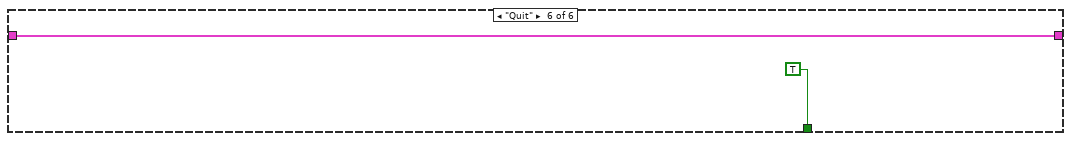
[diagram p11: hidden frame]
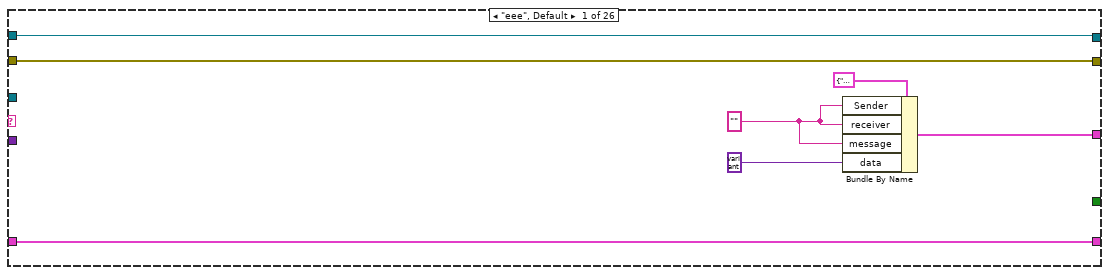
[diagram p13: hidden frame]
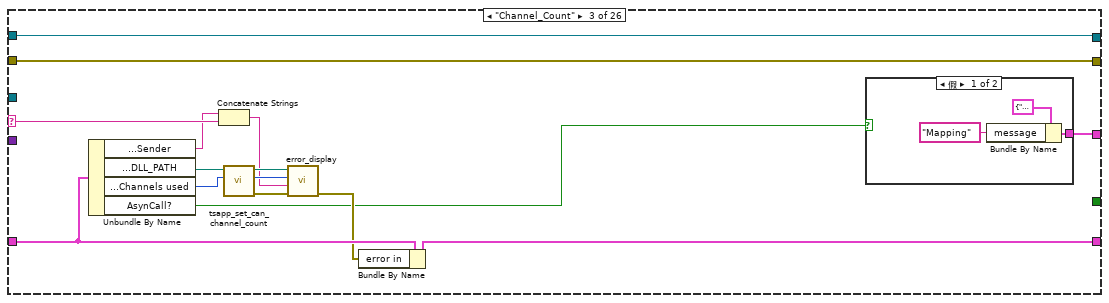
[diagram p14: hidden frame]
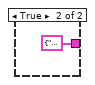
[diagram p15: hidden frame]
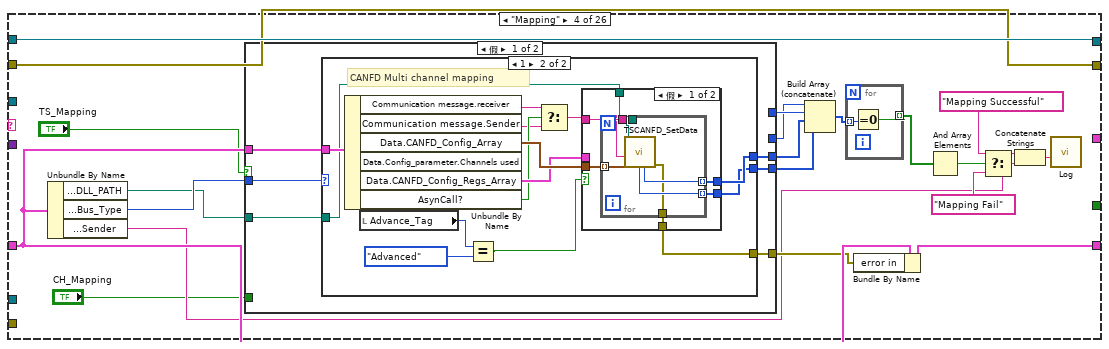
[diagram p16: hidden frame]
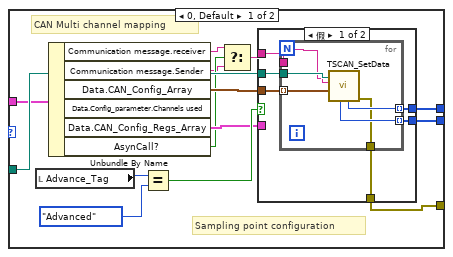
[diagram p17: hidden frame]
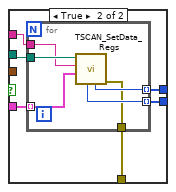
[diagram p18: hidden frame]
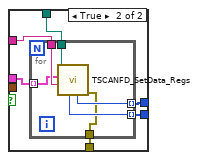
[diagram p19: hidden frame]
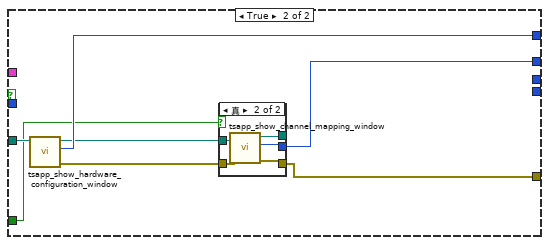
[diagram p20: hidden frame]
diagram:
  n1 = flat-sequence {
    tunnel: [w69] -> w5
    tunnel: [w15] -> w4
    tunnel: [w29] -> w6
    frame #0 {
      w19 = FALSE ("TS_Mapping")
      w27 = FALSE ("Advanced Options")
      w12 = FALSE ("Pause")
      # "Control initialization"
      n2 = Current VI's Path() -> (path=w61:path)
      n3 = local write "Receive Status"(FALSE ("Receive Status")) -> ()
      n4 = local write "Connect ?"(FALSE ("Connect ?")) -> ()
      n5 = Strip Path(path=w61) -> (stripped path=w59:path)  [unwired: 1 out]
      n6 = property on="Data" class="MCListbox (严格)"("ItemNames"=string[][] [] ("项名")) -> ()  [unwired: 2 in, 2 out]
      n7 = Call Chain() -> (call chain=w17:string[])
      n8 = Array Size(array=w17) -> (size(s)=w21:i32)
      n9 = Index Array(array=w17) -> (element=w15:string)  [unwired: 1 in]
      n10 = Greater?(x=w21, y=1) -> (0:w18:bool)
      n11 = property on="窗格" class="Pane"("Origin"=T9 {"Horizontal"=0, "Vertical"=0} ("原点")) -> (error out=w55:errorcluster)  [unwired: 2 in, 1 out]
      n12 = Build Path(base path=w59, name or relative path="data") -> (appended path=w58:path)
      n13 = local write "选项卡控件"(enum32{"Setting", "CAN/CANFD", "DBC_Load"}."Setting" ("选项卡控件")) -> ()
      n14 = call "TSCAN_Configuration_Save.vi"("path"=w58, "error in (no error)"=w55, "Config Name"=w15, "Read/Write"=enum16{"Read", "Write"}."Read") -> ("error in (no error)"=w71:errorcluster, "Data out"=w56:T10)  [unwired: 5 in, 1 out]
      n15 = Unbundle By Name(w56) -> ("Data"=w44:T11)
      n16 = Unbundle By Name(w44) -> ("DBC_Ctr.DBC Path"=w49:path, "DBC_Ctr.DBC loading channel"=w48:i32)
      n17 = Unbundle By Name(w44) -> ("Config_parameter.REC_Channel"=w22:i32, "Config_parameter.Bus_Type"=w52:u16, "Config_parameter.Channels used"=w63:u16, "Config_parameter.DLL_PATH"=w62:path, "Config_parameter.Channel"=w47:i32, "Blf_Log.Blf_Log_PATH"=w31:path)
      n18 = Unbundle By Name(w44) -> ("Send_parameter.SendData"=w68:u8[], "Send_parameter.Data Length"=w67:i32, "Send_parameter.ID"=w66:i32, "Send_parameter.Frame Format"=w65:u8, "Send_parameter.Frame Type"=w64:u8, "Send_parameter.BRS"=w46:enum16{"Close", "Open"}, "Send_parameter.FD Frame"=w45:u8, "Send_parameter.async&sync"=w41:enum16{"async", "sync"}, "Send_parameter.Timeout"=w43:u16)
      n19 = case shown="假" w18 {
        tunnel: [T8."Enabled" ("禁用") T8."Disabled and Grayed Out" ("禁用")] -> w14
        frame False {
        }
        frame True {
        }
      }
      n20 = property on="Diagram shown" class="Bool (严格)"("Visible"=w18) -> ()  [unwired: 2 in, 2 out]
      n21 = local write "BLF_Log_PATH"(w31) -> ()
      n22 = local write "DBC loading channel"(w48) -> ()
      n23 = Bundle By Name(cluster=T10 {"Communication message"={"Sender"="", "receiver"="", "message"="", "data"=variant}, "Data"={"Config_parameter"={"Bus_Type"=0, "Channel"=0, "Channels used"=0, "DLL_PATH"=path "", "Read message type"=0, "REC_Channel"=0}, "Send_parameter"={"SendData"=[], "Data Length"=0, "ID"=0, "Frame Format"=0, "Frame Type"=0, "BRS"=enum."Close", "FD Frame"=0, "async&sync"=enum."async", "Timeout"=0}, "DBC_Ctr"={"DBC Path"=path "", "DBC loading channel"=0, "DatabaseId"=0, "DBMessages"=[], "DBSignals"=[]}, "CAN_Config_Array"=[], "CANFD_Config_Array"=[], "CAN_Config_Regs_Array"=[], "CANFD_Config_Regs_Array"=[], "Blf_Log"={"Blf_Log_PATH"=path ""}, "UDS"={"UDS Control"={"UDS Channel Index"=0, "Request ID"=1992, "Response ID"=2015, "Request ID (Func)"=1, "Session Mode"=1, "Reset Mode"=255, "DTC Mask"=0, "GropOfDTC"=0, "Seed Level"=2, "Seed"=[], "Key Level"=0, "Key"=[], "Read Identifier"=0, "UDS Read Data"=[], "ASCII Data"="", "Write Identifier"=0, "UDS Wrtie Data"=[], "IO Control Identifier"=1, "UDS IOControl Data"=[], "IO Control Mode"=0, "UDS IOControl Read Data"=[], "Routine Control Identifier"=0, "UDS RoutineControl Data"=[], "UDS RoutineControl Read Data"=[], "Routine Control Mode"=1, "SupportFDCAN"=TRUE, "time config"={"p2_timeout"=0, "p2_extended"=0, "s3_servertime"=0, "s3_clienttime"=0}, "ServiceLayer"={"FilledByte"=0, "STMin"=10, "BlockSize"=10, "FCDelay"=10, "MaxLength"=4095}, "Request"=[], "Respond"=[]}, "DiagModuleIndex"=1984}}, "CAN_Buffer"=[], "CANFD_Buffer"=[], "error in"={"status"=FALSE, "code"=0, "source"=""}, "CAN_Period_Datas"=[], "CANFD_period_Datas"=[], "CAN_Filtering_Datas"=[], "CANFD_Filtering_Datas"=[], "AsynCall?"=FALSE} ("Data"), "Communication message.Sender"=w15, "Communication message.receiver"="Receive", "Data"=w44, "AsynCall?"=w18) -> (w69:T10)
      n24 = local write "DBC Path"(w49) -> ()
      n25 = local write "REC_Channel"(w22) -> ()
      n26 = local write "Bus_Type"(w52) -> ()
      n27 = case shown="0, 默认" w52 {
        tunnel: [T8."Disabled and Grayed Out" ("禁用") T8."Enabled" ("禁用")] -> w39
        tunnel: [T8."Enabled" ("禁用") T8."Disabled and Grayed Out" ("禁用")] -> w38
        frame 0, Default {
        }
        frame 1 {
        }
      }
      n28 = local write "Channels used"(w63) -> ()
      n29 = local write "DLL_PATH"(w62) -> ()
      n30 = local write "Channel"(w47) -> ()
      n31 = local write "BRS"(w46) -> ()
      n32 = local write "ID"(w66) -> ()
      n33 = local write "Frame Type"(w64) -> ()
      n34 = local write "FD Frame"(w45) -> ()
      n35 = local write "SendData"(w68) -> ()
      n36 = local write "Data Length"(w67) -> ()
      n37 = local write "Frame Format"(w65) -> ()
      n38 = local write "async&sync"(w41) -> ()
      n39 = local write "Timeout"(w43) -> ()
      n40 = Unbundle By Name(w44) -> ("CAN_Config_Array"=w37:T1[], "CANFD_Config_Array"=w36:T4[], "CAN_Config_Regs_Array"=w35:T6[], "CANFD_Config_Regs_Array"=w34:T5[])
      n41 = property on="DIS_REC" class="Bool (严格)"("DisabledEnum"=w14) -> ()  [unwired: 2 in, 2 out]
      n42 = property on="Config" class="Bool"("DisabledEnum"=w14) -> ()  [unwired: 2 in, 2 out]
      n43 = property on="Connect" class="Bool"("DisabledEnum"=w14) -> ()  [unwired: 2 in, 2 out]
      n44 = property on="STOP" class="Bool"("DisabledEnum"=w14) -> ()  [unwired: 2 in, 2 out]
      n45 = property on="Disconnect" class="Bool"("DisabledEnum"=w14) -> ()  [unwired: 2 in, 2 out]
      n46 = case shown="\"async\", 默认" w41 {
        tunnel: [T8."Disabled and Grayed Out" ("禁用") T8."Enabled" ("禁用")] -> w42
        frame "async", Default {
        }
        frame "sync" {
        }
      }
      n47 = local write "Send_Tag"(enum32{"Single step", "Periodic", "Filter_Pass"}."Single step" ("Send_Tag")) -> ()
      n48 = local write "Advance_Tag"(enum32{"Ordinary", "Advanced"}."Ordinary" ("Advance_Tag")) -> ()
      n49 = local write "Laod BDC Successful?"(FALSE ("Laod BDC Successful?")) -> ()
      n50 = local write "CAN_Config_Array"(w37) -> ()
      n51 = local write "CANFD_Config_Array"(w36) -> ()
      n52 = local write "CANFD_Config_Regs_Array"(w34) -> ()
      n53 = local write "TS_Mapping"(w19) -> ()
      n54 = local write "Diagram shown"(w19) -> ()
      n55 = property on="CAN_Config_Array" class="Arr (严格)"("DisabledEnum"=w38) -> ()  [unwired: 2 in, 2 out]
      n56 = local write "Pause"(w12) -> ()
      n57 = local write "AsynCall"(w12) -> ()
      n58 = local write "CAN_Config_Regs_Array"(w35) -> ()
      n59 = property on="CANFD_Config_Array" class="Arr (严格)"("DisabledEnum"=w39) -> ()  [unwired: 2 in, 2 out]
      n60 = property on="FD Frame" class="Ring (严格)"("DisabledEnum"=w39) -> ()  [unwired: 2 in, 2 out]
      n61 = property on="BRS" class="Enum (严格)"("DisabledEnum"=w39) -> ()  [unwired: 2 in, 2 out]
      n62 = property on="Timeout" class="DigNum (严格)"("DisabledEnum"=w42) -> ()  [unwired: 2 in, 2 out]
      n63 = property on="CANFD_Config_Regs_Array" class="Arr (严格)"("DisabledEnum"=w39) -> ()  [unwired: 2 in, 2 out]
      n64 = property on="CAN_Config_Regs_Array" class="Arr (严格)"("DisabledEnum"=w38) -> ()  [unwired: 2 in, 2 out]
      n65 = local write "Sampling point"(w27) -> ()
      n66 = property on="CH_Mapping" class="Bool (严格)"("DisabledEnum"=T8."Disabled and Grayed Out" ("禁用")) -> ()  [unwired: 2 in, 2 out]
      n67 = local write "DIS_REC"(w27) -> ()
      n68 = property on="log" class="LstBox (严格)"("Item Names"=string[] [] ("项名")) -> (error out=w32:errorcluster)  [unwired: 2 in, 1 out]
      n69 = control-ref of="Tree control"() -> (w30:refnum<vi>)
      n70 = invoke class="Tree (严格)" method="Edit Tree Items.Delete"(reference=w30) -> (error out=w28:errorcluster)  [unwired: 4 in, 4 out]
      n71 = flat-sequence {
        tunnel: w32 -> [_]
        frame #0 {
          n72 = control-ref of="log"() -> (w74:refnum<vi>)
          n73 = call "Log.vi"("Method"=enum16{"Init", "Log"}."Init", "ListBox in"=w74) -> ()  [unwired: 2 in]
        }
      }
      n74 = local write "Fold Data"(FALSE ("Fold Data")) -> ()
      n75 = Merge Errors(w28, w71) -> (w29:errorcluster)
    }
  }
  n76 = flat-sequence {
    tunnel: [w100] -> w11
    tunnel: [w99] -> w10
    tunnel: w6 -> [w94]
    tunnel: w5 -> [w85]
    tunnel: w4 -> [w92]
    tunnel: [w83] -> w2
    tunnel: [w82] -> w1
    frame #0 {
      w96 = ""  # Quit
      n77 = Create User Event(user event datatype=w96) -> (user event=w84:refnum<user-event>)  [unwired: 1 in, 1 out]
      n78 = register-events(w84) -> (reference out=w95:refnum<event-registration>)  [unwired: 2 in, 1 out]
      n79 = Concatenate Strings(w92, "CAN_Data" ("字符串")) -> (w91:string)
      n80 = Obtain Queue(name (unnamed)=w92, element data type=T20 {"Sender"="", "receiver"="", "message"="", "data"=variant} ("Communication message")) -> (queue out=w101:refnum<queue>, error out=w97:errorcluster)  [unwired: 3 in, 1 out]
      n81 = Obtain Queue(name (unnamed)=w91, element data type=T20 {"Sender"="", "receiver"="", "message"="", "data"=variant} ("Communication message")) -> (queue out=w89:refnum<queue>, error out=w88:errorcluster)  [unwired: 3 in, 1 out]
      n82 = while {
        tunnel: w89 -> [w110]
        tunnel: w88 -> [w109]
        tunnel: [w110] -> w87
        tunnel: [w109] -> w86
        shift-right: [w103] -> _
        shift-left: w85 -> [w107]
        i -> [w106]
        stop <- w108 stop-if-true
        # "Receive"
        n83 = Dequeue Element(queue=w110, timeout in ms (-1)=1 ("超时毫秒(-1)"), error in (no error)=w109) -> (element=w113:T20)  [unwired: 3 out]
        n84 = Unbundle By Name(w113) -> ("message"=w112:string, "data"=w111:variant)
        n85 = case shown="\"\"" w112 {
          tunnel: w111 -> [_ _ _ w194 w198 _]
          tunnel: [_ _ _ _ _ TRUE] -> w108
          tunnel: w107 -> [w115 w117 w181 w192 w200 w201]
          tunnel: [w115 w116 w182 w191 w199 w201] -> w104
          frame Default {
          }
          frame "" {
            n86 = local read "Connect ?"() -> (w118:bool)
            n87 = case shown="真" w118 {
              tunnel: [w119 w121] -> w116
              tunnel: w117 -> [w119 w122]
              frame False {
              }
              frame True {
                n88 = case shown="假" "Pause" {
                  tunnel: w122 -> [w137 w178]
                  tunnel: [w127 w178] -> w121
                  frame False {
                    n89 = Unbundle By Name(w137) -> ("Data.Config_parameter.REC_Channel"=w123:i32, "Data.Config_parameter.Bus_Type"=w138:u16)
                    n90 = control-ref of="Data"() -> (w135:refnum<vi>)
                    n91 = case shown="1" w138 {
                      tunnel: w137 -> [w159 w174]
                      tunnel: [w158 w173] -> w136
                      tunnel: w135 -> [w161 w176]
                      tunnel: [w157 w172] -> w134
                      tunnel: [w154 w168] -> w132
                      tunnel: [w153 w167] -> w131
                      tunnel: [w151 w166] -> w129
                      tunnel: [w150 w165] -> w128
                      tunnel: w123 -> [w150 w165]
                      tunnel: [w149 w164] -> w125
                      tunnel: "Fold Data" -> [w148 w163]
                      frame 0, Default {
                        # "CAN_Type"
                        n92 = Unbundle By Name(w159) -> ("Data.Config_parameter.DLL_PATH"=w155:path, "Data.Config_parameter.Read message type"=w162:u16)  [unwired: 1 out]
                        n93 = call "tsfifo_read_can_buffer_frame_count.vi"("AIdxChn"=w150, "路径输入"=w155) -> ("error out"=w156:errorcluster, "ACount out"=w154:i32, "function return"=w153:i32, "路径输出"=w152:path)  [unwired: 6 in]
                        n94 = call "tsfifo_receive_can_msgs.vi"("error in (no error)"=w156, "Read message type"=w162, "AAPPChannel"=w150, "Path"=w152) -> ("error out"=w149:errorcluster, "Return"=w157:i32, "ACANMsgBuffer"=w160:T21, "Path output"=w151:path)  [unwired: 3 in]
                        n95 = call "TSCAN_CAN_Table.vi"("Data输入"=w159, "Fold Data"=w148, "ACANMsgBuffer"=w160, "MCListbox reference handle"=w161) -> ("Data输出"=w158:T10)  [unwired: 7 in]
                      }
                      frame 1 {
                        # "CANFD_Type"
                        n96 = Unbundle By Name(w174) -> ("Data.Config_parameter.DLL_PATH"=w171:path, "Data.Config_parameter.Read message type"=w177:u16)  [unwired: 1 out]
                        n97 = call "tsfifo_read_canfd_buffer_frame_count.vi"("AIdxChn"=w165, "路径输入"=w171) -> ("error out"=w170:errorcluster, "ACount out"=w168:i32, "function return"=w167:i32, "路径输出"=w169:path)  [unwired: 6 in]
                        n98 = call "tsfifo_receive_canfd_msgs.vi"("error in (no error)"=w170, "Display message type"=w177, "AAPPChannel"=w165, "Path"=w169) -> ("error out"=w164:errorcluster, "tsfifo_receive_can_msgs"=w172:i32, "ACANMsgBuffer"=w175:T26, "Path output"=w166:path)  [unwired: 3 in]
                        n99 = call "TSCANfd_CANFD_Table.vi"("Data 3"=w174, "Fold Data"=w163, "ACANMsgBuffer"=w175, "多列列表框输入"=w176) -> ("Data 2"=w173:T10)  [unwired: 7 in]
                      }
                    }
                    "BufferCount" <- w132
                    n100 = disable-structure shown="启用" {
                      disable-tunnel: w129 -> [w147 _]
                      disable-tunnel: w128 -> [w146 _]
                      disable-tunnel: w125 -> [w140 _]
                      disable-tunnel: [w139 _] -> w124
                      frame Enabled {
                        w144 = 0 items=["APP_CAN", "APP_LIN"] ("ABusType")
                        n101 = call "tsapp_get_bus_statistics.vi"("AIdxStat"="AIdxStat", "error in (no error)"=w140, "AIdxChn"=w146, "ABusType"=w144, "路径输入"=w147) -> ("error out"=w139:errorcluster, "AStat"=→"State":dbl, "retuen"=w141:i32)  [unwired: 3 in, 1 out]
                        n102 = Equal To 0?(x=w141) -> (x = 0?=→"Stste?":bool)
                      }
                      frame Disabled {
                      }
                    }
                    n103 = Equal To 0?(x=w134) -> (x = 0?=→"Receive Status":bool)
                    n104 = Equal To 0?(x=w131) -> (x = 0?=→"ok?":bool)
                    n105 = Bundle By Name(cluster=w136, "error in"=w124) -> (w127:T10)
                  }
                  frame True {
                  }
                }
              }
            }
          }
          frame "Clear" {
            n106 = Unbundle By Name(w181) -> ("Data.Config_parameter.Bus_Type"=w180:u16)
            n107 = case shown="0, 默认" w180 {
              tunnel: w181 -> [w185 w188]
              tunnel: [w184 w187] -> w182
              frame 0, Default {
                n108 = Bundle By Name(cluster=w185, "CAN_Buffer"=T21 []) -> (w184:T10)
              }
              frame 1 {
                n109 = Bundle By Name(cluster=w188, "CANFD_Buffer"=T22 []) -> (w187:T10)
              }
            }
            n110 = property on="Data" class="MCListbox (严格)"("ItemNames"=string[][] [] ("项名")) -> ()  [unwired: 2 in, 2 out]
          }
          frame "Config update" {
            n111 = Variant To Data(type=w192, Variant=w194) -> (data=w193:T10, error out=w190:errorcluster)  [unwired: 1 in]
            n112 = Unbundle By Name(w193) -> ("Data"=w189:T11)
            n113 = Bundle By Name(cluster=w192, "Data"=w189, "error in"=w190) -> (w191:T10)
          }
          frame "DBC_Ctr" {
            w195 = T14 {"DBC Path"=path "", "DBC loading channel"=0, "DatabaseId"=0, "DBMessages"=[], "DBSignals"=[]}  # DBC_Ctr
            n114 = Variant To Data(type=w195, Variant=w198) -> (data=w197:T14, error out=w196:errorcluster)  [unwired: 1 in]
            n115 = Bundle By Name(cluster=w200, "Data.DBC_Ctr"=w197, "error in"=w196) -> (w199:T10)
          }
          frame "Quit" {
          }
        }
        n116 = Unbundle By Name(w104) -> ("error in"=w105:errorcluster)
        n117 = call "error_collect.vi"("error in (no error)"=w105) -> ("error IO"=w102:errorcluster)  [unwired: 10 in]
        n118 = Bundle By Name(cluster=w104, "error in"=w102) -> (w103:T10)
        "program loop" <- w106
      }
      n119 = while {
        tunnel: w101 -> [w224]
        tunnel: w97 -> [w223]
        tunnel: [w215] -> w100
        tunnel: [w214] -> w99
        shift-right: [w204] -> _
        shift-left: w85 -> [w210]
        tunnel: w94 -> [_]
        tunnel: w89 -> [w209]
        tunnel: w88 -> [w208]
        tunnel: w84 -> [w207]
        stop <- w213 stop-if-true
        # "Message Handling Loop"
        n120 = Dequeue Element(queue=w224, error in (no error)=w223) -> (queue out=w220:refnum<queue>, element=w222:T20, error out=w219:errorcluster)  [unwired: 1 in, 1 out]
        n121 = Unbundle By Name(w222) -> ("message"=w221:string, "data"=w216:variant)
        n122 = case shown="\"Init\"" w221 {
          selector: w221 -> [_ w240 w278 _ _ _ _ _ _ _ _ _ _ _ _ _ _ _ _ _ _ _ _ _ _ w1223]
          tunnel: [w238 w266 w286 w311 w420 w459 w480 w503 w544 w571 w603 w610 w719 w724 w729 w748 w781 w819 w842 w861 w1151 w1173 w1184 w1212 w1222 w1250] -> w218
          tunnel: w220 -> [w238 w266 w286 w311 w420 w459 w480 w503 w544 w571 w603 w611 w719 w724 w729 w748 w781 w819 w842 w861 w1151 w1173 w1184 w1212 w1222 w1249]
          tunnel: w219 -> [w237 w265 w285 w310 w419 w458 w479 w502 w543 w570 w602 w608 w718 w723 w728 w747 w780 w818 w841 w860 w1150 w1172 w1183 w1211 w1221 w1247]
          tunnel: [w237 w265 w285 w310 w419 w458 w479 w502 w543 w570 w602 w609 w718 w723 w728 w747 w780 w818 w841 w860 w1150 w1172 w1183 w1211 w1221 w1248] -> w217
          tunnel: w216 -> [_ _ _ _ w413 _ w471 w501 _ _ _ w613 _ _ _ _ _ _ _ w851 _ _ _ w1195 w1218 _]
          tunnel: [_ _ _ _ _ _ _ _ _ _ _ _ _ _ _ _ _ _ _ _ _ _ _ _ _ TRUE] -> w213
          tunnel: [w235 w244 w275 _ w415 _ _ _ w534 _ _ w614 _ _ _ _ _ _ _ _ _ _ _ _ _ _] -> w212
          tunnel: [w232 w263 w277 w296 w412 w456 w476 w498 w537 w567 w587 w617 w716 w721 w726 w743 w777 w796 w838 w852 w1147 w1168 w1177 w1199 w1214 w1241] -> w206
          tunnel: w210 -> [w232 w263 w284 w308 w418 w457 w478 w497 w538 w567 w587 w618 w717 w722 w727 w746 w777 w817 w840 w852 w1149 w1171 w1178 w1196 w1220 w1228]
          tunnel: w209 -> [_ _ _ _ _ _ _ _ _ _ _ _ _ _ _ _ w779 w799 w827 _ _ _ _ w1202 _ w1239]
          tunnel: w208 -> [_ _ _ _ _ _ _ _ _ _ _ _ _ _ _ _ w778 w798 w826 _ _ _ _ w1201 _ w1238]
          tunnel: w207 -> [_ _ _ _ _ _ _ _ _ _ _ _ _ _ _ _ _ _ _ _ _ _ _ _ _ w1235]
          frame "eee", Default {
            w233 = ""
            n123 = Bundle By Name(cluster=T20 {"Sender"="", "receiver"="", "message"="", "data"=variant} ("Communication message"), "Sender"=w233, "receiver"=w233, "message"=w233, "data"=variant) -> (w235:T20)
          }
          frame "Init" {
            n124 = Unbundle By Name(w263) -> ("Communication message.Sender"=w239:string, "Data.Config_parameter.DLL_PATH"=w264:path)
            n125 = call "initialize_lib_tsmaster.vi"("AppName"=w239, "Path input"=w264) -> ("error output"=w261:errorcluster, "Path output"=w262:path)  [unwired: 8 in]
            n126 = call "tsapp_disconnect.vi"("error in (no error)"=w261, "Path"=w262) -> ("error output"=w259:errorcluster, "retuen"=w254:i32, "Path output"=w260:path)  [unwired: 7 in]
            n127 = call "Device_Detection.vi"("error in (no error)"=w259, "Path"=w260) -> ("error out"=w257:errorcluster, "retuen"=w253:i32, "Path output"=w258:path)  [unwired: 7 in]
            n128 = call "get_active_application_list.vi"("error in"=w257, "path in"=w258) -> ("error out"=w255:errorcluster, "return"=w252:i32, "path out"=w256:path)  [unwired: 6 in, 1 out]
            n129 = Build Array(w254, w253, w252) -> (w251:i32[])
            n130 = for {
              tunnel: w256 -> [w271]
              tunnel: w255 -> [w270]
              tunnel: w251 -> [w268] mode=indexing
              tunnel: string[] ["tsapp_disconnect", "Device Detection", "get_active_application_list"] -> [w269] mode=indexing
              tunnel: [w267] -> w249 mode=indexing
              n131 = call "error_display.vi"("error in"=w270, "Action name"=w269, "return"=w268, "DLL path"=w271) -> ()  [unwired: 6 in, 2 out]
              n132 = Equal To 0?(x=w268) -> (x = 0?=w267:bool)
            }
            n133 = And Array Elements(Boolean array=w249) -> (logical AND=w248:bool)
            n134 = Select(t="Config Successful", s=w248, f="Config Fail") -> (s? t:f=w245:string)
            n135 = Concatenate Strings(w240, w245) -> (w241:string)
            n136 = call "Log.vi"("Data"=w241) -> ()  [unwired: 3 in]
            n137 = Bundle By Name(cluster=T20 {"Sender"="", "receiver"="", "message"="", "data"=variant} ("Communication message"), "message"="Channel_Count") -> (w244:T20)
          }
          frame "Channel_Count" {
            n138 = Unbundle By Name(w284) -> ("Communication message.Sender"=w272:string, "Data.Config_parameter.DLL_PATH"=w283:path, "Data.Config_parameter.Channels used"=w282:u16, "AsynCall?"=w274:bool)
            n139 = Concatenate Strings(w272, w278) -> (w273:string)
            n140 = call "tsapp_set_can_channel_count.vi"("Aount"=w282, "Path"=w283) -> ("error out"=w279:errorcluster, "return"=w280:i32, "Path output"=w281:path)  [unwired: 7 in]
            n141 = call "error_display.vi"("error in"=w279, "Action name"=w273, "return"=w280, "DLL path"=w281) -> ("error out"=w276:errorcluster)  [unwired: 6 in, 1 out]
            n142 = Bundle By Name(cluster=w284, "error in"=w276) -> (w277:T10)
            n143 = case shown="假" w274 {
              tunnel: [w287 T20 {"Sender"="", "receiver"="", "message"="", "data"=variant} ("Communication message")] -> w275
              frame False {
                n144 = Bundle By Name(cluster=T20 {"Sender"="", "receiver"="", "message"="", "data"=variant} ("Communication message"), "message"="Mapping") -> (w287:T20)
              }
              frame True {
              }
            }
          }
          frame "Mapping" {
            n145 = Unbundle By Name(w308) -> ("Data.Config_parameter.DLL_PATH"=w306:path, "Data.Config_parameter.Bus_Type"=w309:u16, "Communication message.Sender"=w293:string)
            n146 = case shown="假" "TS_Mapping" {
              tunnel: w309 -> [w319 _]
              tunnel: w308 -> [w318 _]
              tunnel: w306 -> [w315 w402]
              tunnel: [w317 _] -> w305
              tunnel: [w316 _] -> w304
              tunnel: [_ w401] -> w297
              tunnel: [w314 w399] -> w295
              tunnel: "CH_Mapping" -> [_ w396]
              tunnel: [_ w398] -> w291
              frame False {
                n147 = case shown="1" w319 {
                  tunnel: w315 -> [w333 w370]
                  tunnel: w318 -> [w332 w371]
                  tunnel: [w326 w364] -> w317
                  tunnel: [w325 w363] -> w316
                  tunnel: [w324 w362] -> w314
                  frame 0, Default {
                    # "Sampling point configuration"
                    # "CAN Multi channel mapping"
                    n148 = local read "Advance_Tag"() -> (w328:enum32{"Ordinary", "Advanced"})
                    n149 = Unbundle By Name(w332) -> ("Communication message.receiver"=w322:string, "Communication message.Sender"=w321:string, "Data.CAN_Config_Array"=w331:T1[], "Data.CAN_Config_Regs_Array"=w329:T6[], "AsynCall?"=w323:bool)  [unwired: 1 out]
                    n150 = Equal?(x=w328, y=enum32{"Ordinary", "Advanced"}."Advanced" ("Advance_Tag")) -> (x = y?=w330:bool)
                    n151 = Select(t=w322, s=w323, f=w321) -> (s? t:f=w320:string)
                    n152 = case shown="假" w330 {
                      tunnel: w333 -> [w339 w351]
                      tunnel: w320 -> [w338 w350]
                      tunnel: w331 -> [w337 _]
                      tunnel: w329 -> [_ w349]
                      tunnel: [w336 w348] -> w326
                      tunnel: [w335 w347] -> w325
                      tunnel: [w334 w346] -> w324
                      frame False {
                        n153 = for {
                          tunnel: w339 -> [w345]
                          tunnel: w338 -> [w344]
                          tunnel: w337 -> [w343] mode=indexing
                          tunnel: [w342] -> w336 mode=indexing
                          tunnel: [w341] -> w335 mode=indexing
                          tunnel: [w340] -> w334
                          n154 = call "TSCAN_SetData.vi"("CAN configuration"=w343, "FAPppName"=w344, "Path"=w345) -> ("error out"=w340:errorcluster, "Config_retuen"=w342:i32, "maping_retuen"=w341:i32)  [unwired: 5 in, 1 out]
                        }
                      }
                      frame True {
                        n155 = for {
                          tunnel: w351 -> [w357]
                          tunnel: w350 -> [w356]
                          tunnel: w349 -> [w355] mode=indexing
                          tunnel: [w354] -> w348 mode=indexing
                          tunnel: [w353] -> w347 mode=indexing
                          tunnel: [w352] -> w346
                          n156 = call "TSCAN_SetData_Regs.vi"("CAN_Config_Regs"=w355, "FAPppName"=w356, "Path"=w357) -> ("error out"=w352:errorcluster, "Config_retuen"=w354:i32, "maping_retuen"=w353:i32)  [unwired: 5 in, 1 out]
                        }
                      }
                    }
                  }
                  frame 1 {
                    # "CANFD Multi channel mapping"
                    n157 = Unbundle By Name(w371) -> ("Communication message.receiver"=w360:string, "Communication message.Sender"=w359:string, "Data.CANFD_Config_Array"=w369:T4[], "Data.CANFD_Config_Regs_Array"=w368:T5[], "AsynCall?"=w361:bool)  [unwired: 1 out]
                    n158 = local read "Advance_Tag"() -> (w367:enum32{"Ordinary", "Advanced"})
                    n159 = Equal?(x=w367, y=enum32{"Ordinary", "Advanced"}."Advanced" ("Advance_Tag")) -> (x = y?=w365:bool)
                    n160 = Select(t=w360, s=w361, f=w359) -> (s? t:f=w358:string)
                    n161 = case shown="假" w365 {
                      tunnel: w370 -> [w377 w387]
                      tunnel: w358 -> [w376 w388]
                      tunnel: w369 -> [w375 _]
                      tunnel: w368 -> [_ w389]
                      tunnel: [w374 w386] -> w364
                      tunnel: [w373 w385] -> w363
                      tunnel: [w372 w384] -> w362
                      frame False {
                        n162 = for {
                          tunnel: w377 -> [w383]
                          tunnel: w376 -> [w382]
                          tunnel: w375 -> [w381] mode=indexing
                          tunnel: [w380] -> w374 mode=indexing
                          tunnel: [w379] -> w373 mode=indexing
                          tunnel: [w378] -> w372
                          n163 = call "TSCANFD_SetData.vi"("AppName"=w382, "CANFD Configuration"=w381, "PATH"=w383) -> ("ERROR OUT"=w378:errorcluster, "configure_baudrate_return"=w380:i32, "mapping_return"=w379:i32)  [unwired: 5 in, 1 out]
                        }
                      }
                      frame True {
                        n164 = for {
                          tunnel: w387 -> [w395]
                          tunnel: w388 -> [w394]
                          tunnel: w389 -> [w393] mode=indexing
                          tunnel: [w392] -> w386 mode=indexing
                          tunnel: [w391] -> w385 mode=indexing
                          tunnel: [w390] -> w384
                          n165 = call "TSCANFD_SetData_Regs.vi"("AppName"=w394, "CANFD_Config_Regs"=w393, "PATH"=w395) -> ("ERROR OUT"=w390:errorcluster, "configure_baudrate_return"=w392:i32, "mapping_return"=w391:i32)  [unwired: 5 in, 1 out]
                        }
                      }
                    }
                  }
                }
              }
              frame True {
                n166 = call "tsapp_show_hardware_configuration_window.vi"("路径输入"=w402) -> ("error out"=w400:errorcluster, "function return"=w401:i32, "路径输出"=w397:path)  [unwired: 8 in]
                n167 = case shown="真" w396 {
                  tunnel: w397 -> [w404 w409]
                  tunnel: w400 -> [w403 w407]
                  tunnel: [w404 w408] -> _
                  tunnel: [_ w405] -> w398
                  tunnel: [w403 w406] -> w399
                  frame False {
                  }
                  frame True {
                    n168 = call "tsapp_show_channel_mapping_window.vi"("error in (no error)"=w407, "路径输入"=w409) -> ("error out"=w406:errorcluster, "function return"=w405:i32, "路径输出"=w408:path)  [unwired: 7 in]
                  }
                }
              }
            }
            n169 = Build Array (concatenate)(w291, w297, w305, w304) -> (w303:i32[])
            n170 = for {
              tunnel: [w313] -> w298 mode=indexing
              tunnel: w303 -> [w312] mode=indexing
              n171 = Equal To 0?(x=w312) -> (x = 0?=w313:bool)
            }
            n172 = Bundle By Name(cluster=w308, "error in"=w295) -> (w296:T10)
            n173 = And Array Elements(Boolean array=w298) -> (logical AND=w302:bool)
            n174 = Select(t="Mapping Successful", s=w302, f="Mapping Fail") -> (s? t:f=w299:string)
            n175 = Concatenate Strings(w293, w299) -> (w294:string)
            n176 = call "Log.vi"("Data"=w294) -> ()  [unwired: 3 in]
          }
          frame "Connect" {
            n177 = Unbundle By Name(w418) -> ("Data.Config_parameter.DLL_PATH"=w417:path, "AsynCall?"=w414:bool)
            n178 = case shown="假" w414 {
              tunnel: w418 -> [w430 w438]
              tunnel: w417 -> [w429 _]
              tunnel: [w430 w438] -> w416
              tunnel: [w425 w435] -> w410
              tunnel: w413 -> [_ w437]
              tunnel: [w424 w434] -> w411
              frame False {
                n179 = call "tsapp_connect.vi"("Path"=w429) -> ("error out"=w428:errorcluster, "retuen"=w427:i32, "Path output"=w431:path)  [unwired: 8 in]
                n180 = Equal To 0?(x=w427) -> (x = 0?=w425:bool)
                n181 = call "tsfifo_enable_receive_fifo.vi"("error in (no error)"=w428, "Path"=w431) -> ("error out"=w424:errorcluster)  [unwired: 8 in, 1 out]
                n182 = case shown="假" w425 {
                  tunnel: ["Conncet  fail" ("消息") "Conncet  Successful" ("消息")] -> w426
                  frame False {
                  }
                  frame True {
                  }
                }
                n183 = call "Log.vi"("Data"=w426) -> ()  [unwired: 3 in]
              }
              frame True {
                n184 = Variant To Data(type=FALSE, Variant=w437) -> (data=w435:bool, error out=w434:errorcluster)  [unwired: 1 in]
              }
            }
            "Connect ?" <- w410
            n185 = Bundle By Name(cluster=w416, "error in"=w411) -> (w412:T10)
            n186 = case shown="真" w410 {
              tunnel: [_ w421] -> w415
              frame False {
              }
              frame True {
                n187 = Bundle By Name(cluster=T20 {"Sender"="", "receiver"="", "message"="", "data"=variant} ("Communication message"), "message"="Clear Buffer") -> (w421:T20)
              }
            }
          }
          frame "Clear Buffer" {
            n188 = Unbundle By Name(w457) -> ("Data.Config_parameter.DLL_PATH"=w439:path, "Data.Config_parameter.Bus_Type"=w455:u16, "Data.Config_parameter.Channel"=w454:i32)
            n189 = case shown="0, 默认" w455 {
              tunnel: w454 -> [w464 w468]
              tunnel: [w463 w467] -> w452
              tunnel: [w462 w466] -> w449
              tunnel: [w461 w465] -> w443
              tunnel: w439 -> [w460 _]
              frame 0, Default {
                n190 = call "tsfifo_clear_can_receive_buffers.vi"("AIdxChn"=w464, "路径输入"=w460) -> ("error out"=w462:errorcluster, "function return"=w463:i32, "路径输出"=w461:path)  [unwired: 7 in]
              }
              frame 1 {
                n191 = call "tsfifo_clear_canfd_receive_buffers.vi"("AIdxChn"=w468) -> ("error out"=w466:errorcluster, "function return"=w467:i32, "路径输出"=w465:path)  [unwired: 8 in]
              }
            }
            n192 = call "tsapp_enable_bus_statistics.vi"("error in (no error)"=w449, "AEnable"=TRUE, "路径输入"=w443) -> ("error out"=w450:errorcluster, "retuen"=w447:i32, "路径输出"=w451:path)  [unwired: 6 in]
            n193 = call "tsapp_clear_bus_statistics.vi"("error in (no error)"=w450, "路径输入"=w451) -> ("error out"=w448:errorcluster, "retuen"=w446:i32)  [unwired: 7 in, 1 out]
            n194 = Equal To 0?(x=w452) -> (x = 0?=w453:bool)
            n195 = Equal To 0?(x=w447) -> (x = 0?=w445:bool)
            n196 = Equal To 0?(x=w446) -> (x = 0?=w444:bool)
            n197 = Bundle By Name(cluster=w457, "error in"=w448) -> (w456:T10)
            n198 = Compound Arithmetic op=AND(w453, w445, w444) -> (w440:bool)
            n199 = case shown="假" w440 {
              tunnel: ["Conncet  fail" ("消息") " Clear Buffer Successful" ("消息")] -> w441
              frame False {
              }
              frame True {
              }
            }
            n200 = call "Log.vi"("Data"=w441) -> ()  [unwired: 3 in]
          }
          frame "Disconnect" {
            n201 = Unbundle By Name(w478) -> ("Data.Config_parameter.DLL_PATH"=w477:path, "AsynCall?"=w472:bool)
            n202 = case shown="假" w472 {
              tunnel: w477 -> [w484 _]
              tunnel: [w483 w485] -> w475
              tunnel: [w481 w486] -> w474
              tunnel: w471 -> [_ w488]
              frame False {
                n203 = call "tsapp_disconnect.vi"("Path"=w484) -> ("error output"=w483:errorcluster, "retuen"=w482:i32)  [unwired: 8 in, 1 out]
                n204 = Equal To 0?(x=w482) -> (x = 0?=w481:bool)
              }
              frame True {
                n205 = Variant To Data(type=FALSE, Variant=w488) -> (data=w486:bool, error out=w485:errorcluster)  [unwired: 1 in]
              }
            }
            n206 = Bundle By Name(cluster=w478, "error in"=w475) -> (w476:T10)
            n207 = case shown="真" w474 {
              tunnel: ["Disonncet  fail" ("消息") "Disonncet  Successful" ("消息")] -> w473
              frame False {
              }
              frame True {
                n208 = local write "Connect ?"(FALSE ("Connect ?")) -> ()
              }
            }
            n209 = call "Log.vi"("Data"=w473) -> ()  [unwired: 3 in]
          }
          frame "DIS_REC" {
            n210 = Variant To Data(type=FALSE, Variant=w501) -> (data=w499:bool, error out=w494:errorcluster)  [unwired: 1 in]
            n211 = Unbundle By Name(w497) -> ("Data.Config_parameter.Bus_Type"=w496:u16, "Data.Config_parameter.DLL_PATH"=w495:path, "Data.Config_parameter.REC_Channel"=w492:i32)
            n212 = case shown="假" w499 {
              tunnel: w496 -> [_ w522]
              tunnel: w495 -> [w507 w520]
              tunnel: w494 -> [w505 w518]
              tunnel: [w506 w517] -> w493
              tunnel: w492 -> [_ w516]
              frame False {
                n213 = call "tsfifo_enable_receive_fifo.vi"("error in (no error)"=w505, "Path"=w507) -> ("error out"=w506:errorcluster)  [unwired: 8 in, 1 out]
                n214 = call "Log.vi"("Data"="EN_REC") -> ()  [unwired: 3 in]
              }
              frame True {
                w514 = "clear_receive_buffers Successful"  # clear_receive_buffers Successful
                n215 = call "tsfifo_disable_receive_fifo.vi"("error in (no error)"=w518, "Path"=w520) -> ("error out"=w519:errorcluster, "Path output"=w521:path)  [unwired: 8 in]
                n216 = case shown="0, 默认" w522 {
                  tunnel: w521 -> [w527 w532]
                  tunnel: w519 -> [w526 w531]
                  tunnel: [w525 w530] -> w517
                  tunnel: w516 -> [w524 w529]
                  tunnel: [w523 w528] -> w512
                  frame 0, Default {
                    n217 = call "tsfifo_clear_can_receive_buffers.vi"("error in (no error)"=w526, "AIdxChn"=w524, "路径输入"=w527) -> ("error out"=w525:errorcluster, "function return"=w523:i32)  [unwired: 6 in, 1 out]
                  }
                  frame 1 {
                    n218 = call "tsfifo_clear_canfd_receive_buffers.vi"("error in (no error)"=w531, "AIdxChn"=w529, "路径输入"=w532) -> ("error out"=w530:errorcluster, "function return"=w528:i32)  [unwired: 6 in, 1 out]
                  }
                }
                n219 = Equal To 0?(x=w512) -> (x = 0?=w515:bool)
                n220 = Select(t=w514, s=w515, f="clear_receive_buffers Fail") -> (s? t:f=w511:string)
                n221 = Concatenate Strings("DIS_REC" ("string"), "\r", w511) -> (w510:string)
                n222 = call "Log.vi"("Data"=w510) -> ()  [unwired: 3 in]
              }
            }
            n223 = Bundle By Name(cluster=w497, "error in"=w493) -> (w498:T10)
          }
          frame "Import" {
            n224 = Read from Binary File(5:w538, 7:"Please select a configuration file" ("对话框窗口（打开现有文件）")) -> (0:w542:errorcluster, 1:w540:bool, 2:w541:T10)  [unwired: 4 in, 1 out]
            n225 = case shown="无错误" w542 {
              selector: w542 -> [_ w562]
              tunnel: w541 -> [w548 _]
              tunnel: w540 -> [w550 _]
              tunnel: w538 -> [w549 w565]
              tunnel: [w547 w565] -> w537
              tunnel: [w546 w559] -> w536
              tunnel: [w545 _] -> w533
              frame No Error {
                n226 = case shown="假" w550 {
                  tunnel: w549 -> [w557 w558]
                  tunnel: w548 -> [w556 _]
                  tunnel: [w554 w558] -> w547
                  tunnel: [w552 _] -> w546
                  tunnel: ["update" ("按钮名称（“确定”）") _] -> w545
                  frame False {
                    w552 = "Import successful" ("消息")
                    n227 = Unbundle By Name(w556) -> ("Data"=w555:T11)
                    n228 = Bundle By Name(cluster=w557, "Data"=w555) -> (w554:T10)
                    n229 = One Button Dialog(message=w552, button name ("OK")="OK" ("按钮名称（“确定”）")) -> ()  [unwired: 1 out]
                  }
                  frame True {
                  }
                }
              }
              frame Error {
                n230 = call <vilib>:"Clear Errors.vi"("error in (no error)"=w562) -> ()  [unwired: 5 in, 2 out]
                n231 = Unbundle By Name(w562) -> ("source"=w563:string)
                n232 = Concatenate Strings("Import Fail" ("消息"), "\r", w563) -> (w559:string)
                n233 = One Button Dialog(message=w559, button name ("OK")="OK" ("按钮名称（“确定”）")) -> ()  [unwired: 1 out]
              }
            }
            n234 = call "Log.vi"("Data"=w536) -> ()  [unwired: 3 in]
            n235 = Bundle By Name(cluster=T20 {"Sender"="", "receiver"="", "message"="", "data"=variant} ("Communication message"), "message"=w533) -> (w534:T20)
          }
          frame "Export" {
            n236 = Write to Binary File(data=w567, 7:"Please edit the configuration name " ("提示（选择或输入文件路径）")) -> (error out=w568:errorcluster)  [unwired: 4 in, 2 out]
            n237 = case shown="无错误" w568 {
              selector: w568 -> [_ w575]
              tunnel: [w572 w574] -> w566
              frame No Error {
                w572 = "Export successful" ("消息")
                n238 = One Button Dialog(message=w572, button name ("OK")="OK" ("按钮名称（“确定”）")) -> ()  [unwired: 1 out]
              }
              frame Error {
                n239 = Unbundle By Name(w575) -> ("source"=w577:string)
                n240 = Concatenate Strings("Export Fail" ("消息"), "\r", w577) -> (w574:string)
                n241 = call <vilib>:"Clear Errors.vi"("error in (no error)"=w575) -> ()  [unwired: 5 in, 2 out]
                n242 = One Button Dialog(message=w574, button name ("OK")="OK" ("按钮名称（“确定”）")) -> ()  [unwired: 1 out]
              }
            }
            n243 = call "Log.vi"("Data"=w566) -> ()  [unwired: 3 in]
          }
          frame "update" {
            n244 = Unbundle By Name(w587) -> ("Data.Config_parameter.Bus_Type"=w601:u16, "Data.Config_parameter.Channel"=w599:i32, "Data.Config_parameter.Channels used"=w600:u16, "Data.Config_parameter.DLL_PATH"=w598:path, "Data.Config_parameter.Read message type"=w597:u16, "Data.Send_parameter.SendData"=w596:u8[], "Data.Send_parameter.Data Length"=w595:i32, "Data.Send_parameter.ID"=w594:i32, "Data.Send_parameter.Frame Format"=w593:u8, "Data.Send_parameter.Frame Type"=w592:u8, "Data.Send_parameter.BRS"=w591:enum16{"Close", "Open"}, "Data.Send_parameter.FD Frame"=w590:u8, "Data.Send_parameter.async&sync"=w589:enum16{"async", "sync"}, "Data.Send_parameter.Timeout"=w588:u16)
            n245 = local write "Bus_Type"(w601) -> ()
            n246 = local write "Channel"(w599) -> ()
            n247 = local write "Channels used"(w600) -> ()
            n248 = local write "DLL_PATH"(w598) -> ()
            n249 = local write "Read message type"(w597) -> ()
            n250 = local write "SendData"(w596) -> ()
            n251 = local write "Data Length"(w595) -> ()
            n252 = local write "ID"(w594) -> ()
            n253 = local write "Frame Format"(w593) -> ()
            n254 = local write "Frame Type"(w592) -> ()
            n255 = local write "BRS"(w591) -> ()
            n256 = local write "FD Frame"(w590) -> ()
            n257 = local write "async&sync"(w589) -> ()
            n258 = local write "Timeout"(w588) -> ()
            n259 = Unbundle By Name(w587) -> ("Data.Blf_Log.Blf_Log_PATH"=w586:path, "Data.CAN_Config_Array"=w584:T1[], "Data.CANFD_Config_Array"=w583:T4[], "Data.CAN_Config_Regs_Array"=w582:T6[], "Data.CANFD_Config_Regs_Array"=w581:T5[], "Data.DBC_Ctr.DBC Path"=w585:path, "Data.DBC_Ctr.DBC loading channel"=w580:i32)
            n260 = local write "BLF_Log_PATH"(w586) -> ()
            n261 = local write "CAN_Config_Array"(w584) -> ()
            n262 = local write "CANFD_Config_Array"(w583) -> ()
            n263 = local write "CAN_Config_Regs_Array"(w582) -> ()
            n264 = local write "CANFD_Config_Regs_Array"(w581) -> ()
            n265 = local write "DBC Path"(w585) -> ()
            n266 = local write "DBC loading channel"(w580) -> ()
          }
          frame "Sending" {
            n267 = Unbundle By Name(w618) -> ("Data.Config_parameter.DLL_PATH"=w619:path, "Data.Config_parameter.Bus_Type"=w620:u16)
            n268 = Variant To Data(type=FALSE, Variant=w613) -> (data=w607:bool)  [unwired: 1 in, 1 out]
            n269 = case shown="1" w620 {
              tunnel: w619 -> [w649 w695]
              tunnel: [w658 w694] -> w617
              tunnel: w618 -> [w658 w694]
              tunnel: [w651 w685] -> w616
              tunnel: [w645 w680] -> w604
              frame 0, Default {
                # "CAN"
                n270 = Unbundle By Name(w658) -> ("Data.Config_parameter.Channel"=w657:i32, "Data.Send_parameter.ID"=w656:i32, "Data.Send_parameter.Frame Format"=w655:u8, "Data.Send_parameter.Frame Type"=w654:u8, "Data.Send_parameter.Data Length"=w653:i32, "Data.Send_parameter.SendData"=w650:u8[], "Data.Send_parameter.async&sync"=w644:enum16{"async", "sync"}, "Data.Send_parameter.Timeout"=w643:u16)
                n271 = Array To Cluster(array=w650) -> (cluster=w652:T27)
                n272 = Bundle By Name(cluster=T23 {"Channel select"=0, "ID"=274, "Frame format"=0, "Frame type"=0, "Length"=3, "Data"={"Data0"=11, "Data1"=0, "Data2"=0, "Data3"=0, "Data4"=0, "Data5"=0, "Data6"=0, "Data7"=0}} ("TCAN"), "Channel select"=w657, "ID"=w656, "Frame format"=w655, "Frame type"=w654, "Length"=w653, "Data"=w652) -> (w660:T23)
                n273 = Tick Count (ms)() -> (millisecond timer value=w646:u32)
                n274 = flat-sequence {
                  tunnel: w660 -> [w666]
                  tunnel: w649 -> [w664]
                  tunnel: [w665] -> w648
                  tunnel: w646 -> [w663]
                  tunnel: [w663] -> w647
                  tunnel: w644 -> [w662]
                  tunnel: w643 -> [w661]
                  tunnel: [w677] -> w651
                  tunnel: w648 -> [w677]
                  tunnel: w647 -> [w675]
                  tunnel: [w674] -> w645
                  frame #0 {
                    n275 = case shown="\"async\", 默认" w662 {
                      tunnel: w666 -> [w669 w672]
                      tunnel: [w668 w671] -> w665
                      tunnel: w664 -> [w667 w673]
                      tunnel: w661 -> [_ w670]
                      frame "async", Default {
                        n276 = call "tsapp_transmit_can_async.vi"("TCAN"=w669, "Path input"=w667) -> ("return"=w668:i32)  [unwired: 7 in, 2 out]
                      }
                      frame "sync" {
                        n277 = call "tsapp_transmit_can_sync.vi"("ATimeoutMS"=w670, "TCAN"=w672, "Path input"=w673) -> ("return"=w671:i32)  [unwired: 6 in, 2 out]
                      }
                    }
                  }
                  frame #1 {
                    n278 = Tick Count (ms)() -> (millisecond timer value=w676:u32)
                    n279 = Subtract(x=w676, y=w675) -> (x-y=w674:u32)
                  }
                }
              }
              frame 1 {
                # "CANFD"
                n280 = Unbundle By Name(w694) -> ("Data.Config_parameter.Channel"=w693:i32, "Data.Send_parameter.ID"=w692:i32, "Data.Send_parameter.Frame Format"=w691:u8, "Data.Send_parameter.Frame Type"=w690:u8, "Data.Send_parameter.Data Length"=w689:i32, "Data.Send_parameter.FD Frame"=w688:u8, "Data.Send_parameter.BRS"=w686:enum16{"Close", "Open"}, "Data.Send_parameter.SendData"=w684:u8[], "Data.Send_parameter.async&sync"=w679:enum16{"async", "sync"}, "Data.Send_parameter.Timeout"=w678:u16)
                n281 = Array To Cluster(array=w684) -> (cluster=w687:T28)
                n282 = Bundle By Name(cluster=T24 {"AIdxchn"=0, "AId"=0, "AIsStd"=0, "BRS"=enum."Close", "AIsData"=0, "ADLC"=0, "AIsFD"=enum."Classic CAN Message", "FDatas"={"Initialize array[0]"=0, "Initialize array[1]"=0, "Initialize array[2]"=0, "Initialize array[3]"=0, "Initialize array[4]"=0, "Initialize array[5]"=0, "Initialize array[6]"=0, "Initialize array[7]"=0, "Initialize array[8]"=0, "Initialize array[9]"=0, "Initialize array[10]"=0, "Initialize array[11]"=0, "Initialize array[12]"=0, "Initialize array[13]"=0, "Initialize array[14]"=0, "Initialize array[15]"=0, "Initialize array[16]"=0, "Initialize array[17]"=0, "Initialize array[18]"=0, "Initialize array[19]"=0, "Initialize array[20]"=0, "Initialize array[21]"=0, "Initialize array[22]"=0, "Initialize array[23]"=0, "Initialize array[24]"=0, "Initialize array[25]"=0, "Initialize array[26]"=0, "Initialize array[27]"=0, "Initialize array[28]"=0, "Initialize array[29]"=0, "Initialize array[30]"=0, "Initialize array[31]"=0, "Initialize array[32]"=0, "Initialize array[33]"=0, "Initialize array[34]"=0, "Initialize array[35]"=0, "Initialize array[36]"=0, "Initialize array[37]"=0, "Initialize array[38]"=0, "Initialize array[39]"=0, "Initialize array[40]"=0, "Initialize array[41]"=0, "Initialize array[42]"=0, "Initialize array[43]"=0, "Initialize array[44]"=0, "Initialize array[45]"=0, "Initialize array[46]"=0, "Initialize array[47]"=0, "Initialize array[48]"=0, "Initialize array[49]"=0, "Initialize array[50]"=0, "Initialize array[51]"=0, "Initialize array[52]"=0, "Initialize array[53]"=0, "Initialize array[54]"=0, "Initialize array[55]"=0, "Initialize array[56]"=0, "Initialize array[57]"=0, "Initialize array[58]"=0, "Initialize array[59]"=0, "Initialize array[60]"=0, "Initialize array[61]"=0, "Initialize array[62]"=0, "Initialize array[63]"=0}} ("TCANFD"), "AIdxchn"=w693, "AId"=w692, "AIsStd"=w691, "AIsData"=w690, "ADLC"=w689, "AIsFD"=w688, "FDatas"=w687, "BRS"=w686) -> (w696:T24)
                n283 = Tick Count (ms)() -> (millisecond timer value=w681:u32)
                n284 = flat-sequence {
                  tunnel: w696 -> [w703]
                  tunnel: w695 -> [w702]
                  tunnel: [w701] -> w683
                  tunnel: w681 -> [w700]
                  tunnel: [w700] -> w682
                  tunnel: w679 -> [w699]
                  tunnel: w678 -> [w698]
                  tunnel: [w714] -> w685
                  tunnel: w683 -> [w714]
                  tunnel: w682 -> [w712]
                  tunnel: [w711] -> w680
                  frame #0 {
                    n285 = case shown="\"async\", 默认" w699 {
                      tunnel: w703 -> [w706 w709]
                      tunnel: w702 -> [w705 w710]
                      tunnel: [w704 w707] -> w701
                      tunnel: w698 -> [_ w708]
                      frame "async", Default {
                        n286 = call "tsapp_transmit_canfd_async.vi"("TCANFD"=w706, "Path"=w705) -> ("return"=w704:i32)  [unwired: 7 in, 2 out]
                      }
                      frame "sync" {
                        n287 = call "tsapp_transmit_canfd_sync.vi"("ATimeoutMS"=w708, "TCANFD"=w709, "Path"=w710) -> ("return"=w707:i32)  [unwired: 6 in, 2 out]
                      }
                    }
                  }
                  frame #1 {
                    n288 = Tick Count (ms)() -> (millisecond timer value=w713:u32)
                    n289 = Subtract(x=w713, y=w712) -> (x-y=w711:u32)
                  }
                }
              }
            }
            "ms" <- w604
            n290 = Wait (ms)(milliseconds to wait=u32 10 ("等待时间（毫秒）")) -> ()  [unwired: 1 out]
            n291 = Equal To 0?(x=w616) -> (x = 0?=→"send successful?":bool)
            n292 = case shown="无错误" w608 {
              selector: w608 -> [w621 w635]
              tunnel: w607 -> [w622 _]
              tunnel: [w622 FALSE] -> w606
              tunnel: w611 -> [w625 w634]
              tunnel: [w624 w633] -> w610
              tunnel: [w623 w632] -> w609
              frame No Error {
                n293 = case shown="真" w622 {
                  tunnel: w625 -> [w629 w631]
                  tunnel: [w628 w631] -> w624
                  tunnel: [w627 w630] -> w623
                  tunnel: w621 -> [w626 w630]
                  frame False {
                    n294 = Flush Queue(queue=w629, error in (no error)=w626) -> (queue out=w628:refnum<queue>, error out=w627:errorcluster)  [unwired: 1 out]
                  }
                  frame True {
                  }
                }
              }
              frame Error {
                n295 = call <vilib>:"Clear Errors.vi"("error in (no error)"=w635) -> ()  [unwired: 5 in, 2 out]
                n296 = Flush Queue(queue=w634) -> (queue out=w633:refnum<queue>, error out=w632:errorcluster)  [unwired: 1 in, 1 out]
              }
            }
            n297 = case shown="真" w606 {
              tunnel: [T20 {"Sender"="", "receiver"="", "message"="", "data"=variant} ("Communication message") w641] -> w614
              frame False {
              }
              frame True {
                n298 = To Variant(anything=TRUE) -> (Variant=w639:variant)
                n299 = Bundle By Name(cluster=T20 {"Sender"="", "receiver"="", "message"="", "data"=variant} ("Communication message"), "message"="Sending", "data"=w639) -> (w641:T20)
              }
            }
          }
          frame "Periodic_Send" {
            n300 = call "TSCAN_Periodic_Sending.vi"("Data"=w717, "Sender"="Periodic_Send") -> ("Data 2"=w716:T10)  [unwired: 9 in]
          }
          frame "Filtering" {
            n301 = call "TSCAN_Receive_Filtering.vi"("Data"=w722, "Sender"="Filtering") -> ("Data 2"=w721:T10)  [unwired: 9 in]
          }
          frame "DBC_Send" {
            n302 = local read "Laod BDC Successful?"() -> (w725:bool)
            n303 = case shown="真" w725 {
              tunnel: w727 -> [w731 w735]
              tunnel: [w731 w732] -> w726
              frame False {
                n304 = One Button Dialog(message="Please load the DBC database first" ("消息")) -> ()  [unwired: 1 in, 1 out]
              }
              frame True {
                n305 = call "TSCAN_DBC_R&S.vi"("Data"=w735, "Sender"="DBC_Send") -> ("Data 2"=w733:T10)  [unwired: 9 in]
                n306 = flat-sequence {
                  tunnel: w733 -> [w736]
                  tunnel: [w736] -> w732
                  frame #0 {
                    n307 = control-ref of="log"() -> (w737:refnum<vi>)
                    n308 = call "Log.vi"("Method"=enum16{"Init", "Log"}."Init", "ListBox in"=w737) -> ()  [unwired: 2 in]
                  }
                }
              }
            }
          }
          frame "UDS" {
            n309 = Format Date/Time String() -> (date/time string=w742:string)  [unwired: 3 in]
            n310 = Concatenate Strings("UDS" ("Sender"), w742) -> (w740:string)
            n311 = local read "Connect ?"() -> (w745:bool)
            n312 = case shown="真" w745 {
              tunnel: w746 -> [w753 w757]
              tunnel: [w753 w754] -> w744
              tunnel: w740 -> [_ w756]
              tunnel: "AsynCall" -> [_ w755]
              frame False {
                n313 = One Button Dialog(message="Please connect the device first" ("消息")) -> ()  [unwired: 1 in, 1 out]
              }
              frame True {
                n314 = case shown="真" w755 {
                  tunnel: w757 -> [w759 w761]
                  tunnel: w756 -> [w760 w762]
                  tunnel: [w758 w761] -> w754
                  frame False {
                    n315 = call "TSCAN_UDS.vi"("Data"=w759, "Sender"=w760) -> ("Data out"=w758:T10)  [unwired: 9 in]
                  }
                  frame True {
                    n316 = vi-ref "TSCAN_UDS.vi"() -> (w764:refnum<vi>)
                    n317 = property class="VI"(reference=w764) -> (error out=w768:errorcluster, "Name"=w763:string)  [unwired: 1 in, 1 out]
                    n318 = Open VI Reference(type specifier VI Refnum (for type only)=refnum<vi> refnum ("类型说明符VI引用句柄（仅用于类型）"), vi path=w763, options=128 ("选项"), error in (no error)=w768) -> (vi reference=w766:refnum<vi>, error out=w767:errorcluster)  [unwired: 2 in]
                    n319 = call-by-ref "?"(reference=w766, error in=w767, "Data"=w761, "Sender"=w762) -> ()  [unwired: 9 in, 3 out]
                  }
                }
              }
            }
            n320 = flat-sequence {
              tunnel: w744 -> [w749]
              tunnel: [w749] -> w743
              frame #0 {
                n321 = control-ref of="log"() -> (w750:refnum<vi>)
                n322 = call "Log.vi"("Method"=enum16{"Init", "Log"}."Init", "ListBox in"=w750) -> ()  [unwired: 2 in]
              }
            }
          }
          frame "Clear" {
            n323 = Unbundle By Name(w777) -> ("Data.Config_parameter.Bus_Type"=w776:u16, "Data.Config_parameter.DLL_PATH"=w775:path)
            n324 = local read "REC_Channel"() -> (w770:i32)
            n325 = case shown="0, 默认" w776 {
              tunnel: w775 -> [w789 w792]
              tunnel: w770 -> [w788 w791]
              tunnel: [w787 w790] -> w771
              frame 0, Default {
                n326 = call "tsfifo_clear_can_receive_buffers.vi"("AIdxChn"=w788, "路径输入"=w789) -> ("function return"=w787:i32)  [unwired: 7 in, 2 out]
              }
              frame 1 {
                n327 = call "tsfifo_clear_canfd_receive_buffers.vi"("AIdxChn"=w791, "路径输入"=w792) -> ("function return"=w790:i32)  [unwired: 7 in, 2 out]
              }
            }
            n328 = Bundle By Name(cluster=T20 {"Sender"="", "receiver"="", "message"="", "data"=variant} ("Communication message"), "message"="Clear") -> (w773:T20)
            n329 = disable-structure shown="启用" {
              disable-tunnel: w771 -> [w784 _]
              frame Enabled {
                n330 = Equal To 0?(x=w784) -> (x = 0?=w783:bool)
                n331 = case shown="真" w783 {
                  tunnel: ["Clear  fail" ("消息") "Clear  Successful" ("消息")] -> w782
                  frame False {
                  }
                  frame True {
                  }
                }
                n332 = call "Log.vi"("Data"=w782) -> ()  [unwired: 3 in]
              }
              frame Disabled {
              }
            }
            n333 = Enqueue Element(queue=w779, element=w773, error in (no error)=w778) -> ()  [unwired: 1 in, 3 out]
          }
          frame "Load_DBC" {
            n334 = Unbundle By Name(w817) -> ("Data.Config_parameter.DLL_PATH"=w814:path, "Data.DBC_Ctr.DBC Path"=w813:path, "Data.DBC_Ctr.DBC loading channel"=w816:i32)
            n335 = Build Array(w816) -> (w815:i32[])
            n336 = control-ref of="Tree control"() -> (w811:refnum<vi>)
            n337 = call "TSCAN_LoadCANDBC.vi"("ABindChannels"=w815, "ADBCAbsolutePath"=w813, "Path"=w814) -> ("error out"=w808:errorcluster, "AIdOut"=w806:u32, "return"=w812:i32, "Path output"=w810:path)  [unwired: 5 in]
            n338 = Equal To 0?(x=w812) -> (x = 0?=w805:bool)
            "Laod BDC Successful?" <- w805
            n339 = case shown="假" w805 {
              tunnel: [w820 w821] -> w809
              frame False {
                w820 = "Load DBC Fail" ("消息")
                n340 = One Button Dialog(message=w820) -> ()  [unwired: 1 in, 1 out]
              }
              frame True {
                w821 = "Load DBC Succeful" ("消息")
                n341 = One Button Dialog(message=w821) -> ()  [unwired: 1 in, 1 out]
              }
            }
            n342 = call "TSCAN_GetDBCTable.vi"("error in"=w808, "ADatabaseId"=w806, "path in"=w810) -> ("error out"=w795:errorcluster, "DBNode"=w794:T29, "DBSignals"=w803:T25, "DBMessages"=w804:T15[], "NetworkName"=w793:string)  [unwired: 3 in, 1 out]
            n343 = call "DBTableToTree.vi"("NetworkName"=w793, "error in (no error)"=w795, "DBNode"=w794, "DBSignals"=w803, "reference"=w811) -> ("error out"=w807:errorcluster)  [unwired: 6 in]
            n344 = Bundle By Name(cluster=w817, "error in"=w807, "Data.DBC_Ctr.DatabaseId"=w806, "Data.DBC_Ctr.DBMessages"=w804, "Data.DBC_Ctr.DBSignals"=w803) -> (w796:T10)
            n345 = call "Log.vi"("Data"=w809) -> ()  [unwired: 3 in]
            n346 = To Variant(anything=w796) -> (Variant=w797:variant)
            n347 = Bundle By Name(cluster=T20 {"Sender"="", "receiver"="", "message"="", "data"=variant} ("元素"), "message"="Config update" ("Communication message.message"), "data"=w797) -> (w800:T20)
            n348 = Enqueue Element(queue=w799, element=w800, error in (no error)=w798) -> ()  [unwired: 1 in, 3 out]
          }
          frame "Unload_DBC" {
            n349 = Unbundle By Name(w840) -> ("Data.Config_parameter.DLL_PATH"=w839:path)
            n350 = call "tsdb_unload_can_dbs.vi"("path"=w839) -> ("错误输出"=w837:errorcluster, "Return Type"=w836:i32)  [unwired: 8 in, 1 out]
            n351 = Equal To 0?(x=w836) -> (x = 0?=w835:bool)
            n352 = Bundle By Name(cluster=w840, "Data.DBC_Ctr.DatabaseId"=u32 0, "Data.DBC_Ctr.DBMessages"=T15[] [], "Data.DBC_Ctr.DBSignals"=T25 []) -> (w825:T10)
            n353 = case shown="真" w835 {
              tunnel: [w843 w847] -> w834
              tunnel: [_ w845] -> w832
              frame False {
                w843 = "Unload DBC Fail" ("消息")
                n354 = One Button Dialog(message=w843) -> ()  [unwired: 1 in, 1 out]
              }
              frame True {
                w847 = "Unload DBC Succeful" ("消息")
                n355 = control-ref of="Tree control"() -> (w846:refnum<vi>)
                n356 = local write "Laod BDC Successful?"(FALSE ("Laod BDC Successful?")) -> ()
                n357 = invoke class="Tree (严格)" method="Edit Tree Items.Delete"(reference=w846) -> (error out=w845:errorcluster)  [unwired: 4 in, 4 out]
                n358 = One Button Dialog(message=w847) -> ()  [unwired: 1 in, 1 out]
              }
            }
            n359 = To Variant(anything=w825) -> (Variant=w828:variant)
            n360 = Bundle By Name(cluster=T20 {"Sender"="", "receiver"="", "message"="", "data"=variant} ("元素"), "message"="Config update" ("Communication message.message"), "data"=w828) -> (w829:T20)
            n361 = Merge Errors(w832, w837) -> (w833:errorcluster)
            n362 = call "Log.vi"("Data"=w834) -> ()  [unwired: 3 in]
            n363 = Enqueue Element(queue=w827, element=w829, error in (no error)=w826) -> ()  [unwired: 1 in, 3 out]
            n364 = Bundle By Name(cluster=w825, "error in"=w833) -> (w838:T10)
          }
          frame "DBC_Define" {
            n365 = Variant To Data(type=refnum<vi> refnum ("CtlRef"), Variant=w851) -> (data=w849:refnum<vi>)  [unwired: 1 in, 1 out]
            n366 = property class="Tree (严格)"(reference=w849) -> (reference out=w859:refnum<vi>, error out=w854:errorcluster, "Value"=w848:string)  [unwired: 1 in]
            n367 = invoke class="Tree (严格)" method="Navigate Tree.Get Parent"(reference=w859, error in=w854, "tag"=w848) -> (reference out=w858:refnum<vi>, error out=w853:errorcluster, "Navigate Tree:Get Parent"=w855:string)  [unwired: 1 in, 1 out]
            n368 = xnode "匹配正则表达式"("输入字符串"=w855, "正则表达式"="_[0-9]+$" ("regular expression")) -> ("匹配之前"=w856:string)  [unwired: 4 in, 4 out]
            n369 = case shown="默认" w856 {
              selector: w856 -> [w980 _]
              tunnel: w852 -> [w985 w1020]
              tunnel: w848 -> [w983 w1015]
              tunnel: w858 -> [w989 _]
              tunnel: w855 -> [w981 _]
              tunnel: w853 -> [w979 _]
              frame Default {
                n370 = invoke class="Tree (严格)" method="Navigate Tree.Get Parent"(reference=w989, error in=w979, "tag"=w981) -> (error out=w982:errorcluster, "Navigate Tree:Get Parent"=w988:string)  [unwired: 1 in, 2 out]
                n371 = Unbundle By Name(w985) -> ("Data.DBC_Ctr.DBSignals"=w984:T25)
                n372 = Equal?(x=w988, y="Messages") -> (x = y?=w986:bool)
                n373 = call <vilib>:"Clear Errors.vi"("error in (no error)"=w982) -> ()  [unwired: 5 in, 2 out]
                n374 = case shown="真" w986 {
                  tunnel: w984 -> [_ w999]
                  tunnel: w980 -> [_ w998]
                  tunnel: w983 -> [_ w996]
                  frame False {
                  }
                  frame True {
                    n375 = for {
                      tunnel: w999 -> [w1008] mode=indexing
                      tunnel: w998 -> [w1006]
                      tunnel: [w1004] -> w997
                      stop <- w1005 stop-if-true
                      n376 = Unbundle By Name(w1008) -> ("SignalList"=w1004:T16[], "MessageName"=w1007:string)
                      n377 = Equal?(x=w1007, y=w1006) -> (x = y?=w1005:bool)
                    }
                    n378 = control-ref of="DBC Tab"() -> (w990:refnum<vi>)
                    n379 = control-ref of="Signal Table"() -> (w991:refnum<vi>)
                    n380 = property on="Property Node" class="Tbl (严格)"(reference=w991) -> ("Value"=w994:string[][])  [unwired: 1 in, 2 out]
                    n381 = for {
                      tunnel: w997 -> [w1000] mode=indexing
                      tunnel: w996 -> [w1002]
                      tunnel: [w1000] -> w995
                      stop <- w1001 stop-if-true
                      n382 = Unbundle By Name(w1000) -> ("Name"=w1003:string)
                      n383 = Equal?(x=w1003, y=w1002) -> (x = y?=w1001:bool)
                    }
                    n384 = property on="Property Node" class="TabCtl (严格)"(reference=w990, "Value"=enum32{"Message", "Signal"}."Signal" ("Tab Control 2")) -> ()  [unwired: 1 in, 2 out]
                    n385 = call "Signal analysis.vi"("DBSignal"=w995, "Value in"=w994) -> ("Value out"=w993:string[][])  [unwired: 9 in]
                    n386 = property on="Property Node" class="Tbl (严格)"(reference=w991, "Value"=w993) -> ()  [unwired: 1 in, 2 out]
                  }
                }
              }
              frame "Messages", "RX Message", "TX Message" {
                n387 = Unbundle By Name(w1020) -> ("Data.DBC_Ctr.DBMessages"=w1019:T15[])
                n388 = control-ref of="Message Table"() -> (w1009:refnum<vi>)
                n389 = xnode "Match Regular Expression"("输入字符串"=w1015, "正则表达式"="_[0-9]+$" ("regular expression")) -> ("匹配之前"=w1014:string)  [unwired: 4 in, 4 out]
                n390 = for {
                  tunnel: w1019 -> [w1138] mode=indexing
                  tunnel: w1014 -> [w1140]
                  tunnel: [w1138] -> w1018
                  stop <- w1139 stop-if-true
                  n391 = Unbundle By Name(w1138) -> ("Name"=w1141:string)
                  n392 = Equal?(x=w1141, y=w1140) -> (x = y?=w1139:bool)
                }
                n393 = property on="Property Node" class="Tbl (严格)"(reference=w1009) -> (error out=w1010:errorcluster, "Value"=w1017:string[][])  [unwired: 1 in, 1 out]
                n394 = control-ref of="DBC Tab"() -> (w1011:refnum<vi>)
                n395 = call "Message analysis.vi"("DBMessage"=w1018, "Value in"=w1017) -> ("Value out"=w1016:string[][])  [unwired: 9 in]
                n396 = property on="Property Node" class="Tbl (严格)"(reference=w1009, error in=w1010, "Value"=w1016) -> ()  [unwired: 2 out]
                n397 = property on="Property Node" class="TabCtl (严格)"(reference=w1011, "Value"=enum32{"Message", "Signal"}."Message" ("Tab Control 2")) -> ()  [unwired: 1 in, 2 out]
              }
            }
          }
          frame "GetCount_DBC" {
            n398 = Unbundle By Name(w1149) -> ("Data.Config_parameter.DLL_PATH"=w1148:path)
            n399 = call "tsdb_get_can_db_count.vi"("路径输入"=w1148) -> ("error out"=w1146:errorcluster, "ACount out"=w1143:i32, "return"=w1145:i32)  [unwired: 7 in, 1 out]
            n400 = Equal To 0?(x=w1145) -> (x = 0?=w1144:bool)
            n401 = case shown="真" w1144 {
              tunnel: w1143 -> [_ w1158]
              tunnel: [w1153 w1156] -> w1142
              frame False {
                n402 = call <vilib>:"Space Constant.vi"() -> ("String"=w1154:string)
                n403 = Concatenate Strings("GetCount", w1154, "Fail" ("字符串")) -> (w1153:string)
              }
              frame True {
                n404 = Number To Decimal String(number=w1158) -> (decimal integer string=w1157:string)  [unwired: 1 in]
                n405 = call <vilib>:"Space Constant.vi"() -> ("String"=w1159:string)
                n406 = Concatenate Strings("GetCount", w1159, w1157) -> (w1156:string)
              }
            }
            n407 = Bundle By Name(cluster=w1149, "error in"=w1146) -> (w1147:T10)
            n408 = call "Log.vi"("Data"=w1142) -> ()  [unwired: 3 in]
          }
          frame "Start Log" {
            n409 = Unbundle By Name(w1171) -> ("Data.Config_parameter.DLL_PATH"=w1170:path, "Data.Blf_Log.Blf_Log_PATH"=w1161:path)
            n410 = Path To String(path=w1161) -> (string=w1162:string)
            n411 = call "tsapp_start_logging.vi"("AFullFileName"=w1162, "路径输入"=w1170) -> ("error out"=w1167:errorcluster, "retuen"=w1169:i32)  [unwired: 7 in, 1 out]
            n412 = Equal To 0?(x=w1169) -> (x = 0?=w1166:bool)
            n413 = Select(t=" Start Log Successful ", s=w1166, f=" Start Log Fail ") -> (s? t:f=w1163:string)
            n414 = Bundle By Name(cluster=w1171, "error in"=w1167) -> (w1168:T10)
            n415 = call "Log.vi"("Data"=w1163) -> ()  [unwired: 3 in]
          }
          frame "Stop Log" {
            n416 = Unbundle By Name(w1178) -> ("Data.Config_parameter.DLL_PATH"=w1176:path)
            n417 = call "tsapp_stop_logging.vi"("Path"=w1176) -> ("error out"=w1174:errorcluster, "retuen"=w1175:i32)  [unwired: 8 in, 1 out]
            n418 = Equal To 0?(x=w1175) -> (x = 0?=w1182:bool)
            n419 = Select(t=" Stop Log Successful ", s=w1182, f=" Stop Log Fail ") -> (s? t:f=w1179:string)
            n420 = Bundle By Name(cluster=w1178, "error in"=w1174) -> (w1177:T10)
            n421 = call "Log.vi"("Data"=w1179) -> ()  [unwired: 3 in]
          }
          frame "Config update" {
            n422 = Variant To Data(type=w1196, Variant=w1195) -> (data=w1194:T10, error out=w1204:errorcluster)  [unwired: 1 in]
            n423 = Unbundle By Name(w1194) -> ("Data.Config_parameter"=w1192:T12, "Data.Send_parameter"=w1191:T13, "Data.DBC_Ctr"=w1190:T14, "Data.CAN_Config_Array"=w1189:T1[], "Data.CANFD_Config_Array"=w1188:T4[], "Data.CAN_Config_Regs_Array"=w1187:T6[], "Data.CANFD_Config_Regs_Array"=w1186:T5[], "Data.Blf_Log"=w1185:T17)
            n424 = Bundle By Name(cluster=w1196, "Data.Config_parameter"=w1192, "Data.Send_parameter"=w1191, "Data.DBC_Ctr"=w1190, "Data.CAN_Config_Array"=w1189, "Data.CANFD_Config_Array"=w1188, "Data.CAN_Config_Regs_Array"=w1187, "Data.CANFD_Config_Regs_Array"=w1186, "Data.Blf_Log"=w1185) -> (w1193:T10)
            n425 = Current VI's Path() -> (path=w1208:path)
            n426 = Strip Path(path=w1208) -> (stripped path=w1206:path)  [unwired: 1 out]
            n427 = Unbundle By Name(w1193) -> ("Communication message.Sender"=w1210:string)
            n428 = Bundle By Name(cluster=T20 {"Sender"="", "receiver"="", "message"="", "data"=variant} ("元素"), "message"="Config update" ("Communication message.message"), "data"=w1195) -> (w1197:T20)
            n429 = Build Path(base path=w1206, name or relative path="data") -> (appended path=w1205:path)
            n430 = Enqueue Element(queue=w1202, element=w1197, error in (no error)=w1201) -> ()  [unwired: 1 in, 3 out]
            n431 = call "TSCAN_Configuration_Save.vi"("path"=w1205, "error in (no error)"=w1204, "Config Name"=w1210, "Read/Write"=enum16{"Read", "Write"}."Write", "Data"=w1193) -> ("error in (no error)"=w1203:errorcluster)  [unwired: 4 in, 2 out]
            n432 = Bundle By Name(cluster=w1193, "error in"=w1203) -> (w1199:T10)
          }
          frame "Diagram shown" {
            n433 = Variant To Data(type=FALSE, Variant=w1218) -> (data=w1216:bool, error out=w1215:errorcluster)  [unwired: 1 in]
            n434 = control-ref of="本VI"() -> (w1219:refnum<vi>)
            n435 = property on="Property Node" class="VI"(reference=w1219, error in=w1215, "BDWin.Open"=w1216) -> (error out=w1213:errorcluster)  [unwired: 1 out]
            n436 = Bundle By Name(cluster=w1220, "error in"=w1213) -> (w1214:T10)
          }
          frame "Quit" {
            n437 = Bundle By Name(cluster=w1228, "Data.DBC_Ctr.DatabaseId"=u32 0, "Data.DBC_Ctr.DBMessages"=T15[] [], "Data.DBC_Ctr.DBSignals"=T25 []) -> (w1224:T10)
            n438 = Generate User Event(user event=w1235, event data cluster=w1223) -> ()  [unwired: 2 in, 2 out]
            n439 = Bundle By Name(cluster=T20 {"Sender"="", "receiver"="", "message"="", "data"=variant} ("元素"), "message"=w1223) -> (w1236:T20)
            n440 = Enqueue Element(queue=w1239, element=w1236, error in (no error)=w1238) -> (error out=w1225:errorcluster)  [unwired: 1 in, 2 out]
            n441 = flat-sequence {
              tunnel: w1225 -> [_]
              frame #0 {
                n442 = Wait (ms)(milliseconds to wait=u32 50 ("等待时间（毫秒）")) -> ()  [unwired: 1 out]
              }
            }
            n443 = Current VI's Path() -> (path=w1245:path)
            n444 = Unbundle By Name(w1224) -> ("Communication message.Sender"=w1227:string, "Data.Config_parameter.DLL_PATH"=w1233:path, "AsynCall?"=w1226:bool)
            n445 = Strip Path(path=w1245) -> (stripped path=w1243:path)  [unwired: 1 out]
            n446 = Build Path(base path=w1243, name or relative path="data") -> (appended path=w1242:path)
            n447 = case shown="假" w1226 {
              tunnel: w1233 -> [w1256 _]
              tunnel: [w1253 _] -> w1232
              frame False {
                n448 = call "tsapp_disconnect.vi"("Path"=w1256) -> ("error output"=w1255:errorcluster, "Path output"=w1254:path)  [unwired: 8 in, 1 out]
                n449 = call "finalize_lib_tsmaster.vi"("error in (no error)"=w1255, "Path"=w1254) -> ("error out"=w1253:errorcluster)  [unwired: 8 in, 1 out]
              }
              frame True {
              }
            }
            n450 = call "TSCAN_Configuration_Save.vi"("path"=w1242, "Config Name"=w1227, "Read/Write"=enum16{"Read", "Write"}."Write", "Data"=w1224) -> ("error in (no error)"=w1240:errorcluster)  [unwired: 5 in, 2 out]
            n451 = Flush Queue(queue=w1249, error in (no error)=w1247) -> (queue out=w1250:refnum<queue>, error out=w1248:errorcluster)  [unwired: 1 out]
            n452 = Merge Errors(w1240, w1232) -> (w1234:errorcluster)
            n453 = Bundle By Name(cluster=w1228, "error in"=w1234) -> (w1241:T10)
          }
        }
        n454 = Unbundle By Name(w206) -> ("error in"=w205:errorcluster)
        n455 = Unbundle By Name(w212) -> ("message"=w211:string)
        n456 = call "error_collect.vi"("error in (no error)"=w205) -> ("error IO"=w203:errorcluster)  [unwired: 10 in]
        n457 = case shown="\"default\", 默认" w211 {
          tunnel: w218 -> [w229 w231]
          tunnel: w217 -> [w228 w230]
          tunnel: w212 -> [w227 _]
          tunnel: [w226 w231] -> w215
          tunnel: [w225 w230] -> w214
          frame "default", Default {
            n458 = Enqueue Element(queue=w229, element=w227, error in (no error)=w228) -> (queue out=w226:refnum<queue>, error out=w225:errorcluster)  [unwired: 1 in, 1 out]
          }
          frame "" {
          }
        }
        n459 = Bundle By Name(cluster=w206, "error in"=w203) -> (w204:T10)
      }
      n460 = while {
        tunnel: w101 -> [w1266]
        tunnel: w97 -> [w1264]
        tunnel: w92 -> [w1260]
        tunnel: w95 -> [w1259]
        tunnel: [w1258] -> w83
        tunnel: w84 -> [w1257]
        tunnel: [w1257] -> w82
        stop <- w1267 stop-if-true
        # "Event Handling Loop"
        n461 = event shown="[1] \"DLL_PATH\", \"Bus_Type\", \"Channels used\", \"Read message type\", \"Channel\", \"SendData\", \"Data Length\", \"ID\", \"Frame Format\", \"Frame Type\", \"BRS\", \"FD Frame\", \"DBC Path\", \"DBC loading channel\", \"CAN_Config_Array\", \"CANFD_Config_Array\", \"async&sync\", \"Timeout\", \"CAN_Config_Regs_Array\", \"CANFD_Config_Regs_Array\", \"BLF_Log_PATH\", \"REC_Channel\": 值改变" {
          selector: w1259 -> [_ _ _ _ _ _ _ _ _ _ _ _ _ _ _ _ _ _ _ _ _ _ _ _ _ _]
          dyn-events: [_ _ _ _ _ _ _ _ _ _ _ _ _ _ _ _ _ _ _ _ _ _ _ _ _ _] -> w1258
          timeout: _ -> [_ _ _ _ _ _ _ _ _ _ _ _ _ _ _ _ _ _ _ _ _ _ _ _ _ _]
          tunnel: [_ _ _ _ _ _ _ _ _ _ _ _ _ _ _ _ _ _ _ _ _ _ _ w1437 w1445 TRUE ("放弃？")] -> w1267
          tunnel: w1266 -> [w1277 w1313 w1326 w1331 w1335 w1342 w1347 w1351 w1361 w1366 w1371 w1378 w1383 w1388 w1393 w1398 w1403 w1408 w1413 w1420 w1425 w1430 w1435 w1440 w1444 w1449]
          tunnel: [w1277 w1313 w1326 w1331 w1335 w1342 w1347 w1351 w1361 w1366 w1371 w1378 w1383 w1388 w1393 w1398 w1403 w1408 w1413 w1420 w1425 w1430 w1435 w1440 w1442 w1447] -> w1265
          tunnel: [T20 {"Sender"="", "receiver"="", "message"="", "data"=variant} ("Communication message") w1310 w1322 w1329 _ w1339 w1344 _ w1357 w1363 w1368 w1375 w1380 w1385 w1390 w1394 w1399 w1405 w1410 w1416 w1422 w1427 w1432 _ _ _] -> w1262
          tunnel: [w1276 w1279 w1325 w1327 w1332 w1338 w1343 w1350 w1360 w1362 w1367 w1372 w1379 w1384 w1389 w1397 w1402 w1404 w1409 w1419 w1421 w1426 w1431 w1436 w1441 w1446] -> w1263
          tunnel: w1264 -> [w1276 w1279 w1325 w1327 w1332 w1338 w1343 w1350 w1360 w1362 w1367 w1372 w1379 w1384 w1389 w1397 w1402 w1404 w1409 w1419 w1421 w1426 w1431 w1436 w1441 w1446]
          tunnel: w1260 -> [_ _ _ _ _ _ _ _ _ _ _ _ _ _ _ _ _ _ _ _ _ _ _ _ _ _]
          event Timeout {
            n462 = event-data() -> ()  [unwired: 1 in, 3 out]
          }
          event "DLL_PATH", "Bus_Type", "Channels used", "Read message type", "Channel", "SendData", "Data Length", "ID", "Frame Format", "Frame Type", "BRS", "FD Frame", "DBC Path", "DBC loading channel", "CAN_Config_Array", "CANFD_Config_Array", "async&sync", "Timeout", "CAN_Config_Regs_Array", "CANFD_Config_Regs_Array", "BLF_Log_PATH", "REC_Channel": Value Change {
            n463 = event-data() -> ()  [unwired: 1 in, 1 out]
            n464 = Bundle By Name(cluster=T10 {"Communication message"={"Sender"="", "receiver"="", "message"="", "data"=variant}, "Data"={"Config_parameter"={"Bus_Type"=0, "Channel"=0, "Channels used"=0, "DLL_PATH"=path "", "Read message type"=0, "REC_Channel"=0}, "Send_parameter"={"SendData"=[], "Data Length"=0, "ID"=0, "Frame Format"=0, "Frame Type"=0, "BRS"=enum."Close", "FD Frame"=0, "async&sync"=enum."async", "Timeout"=0}, "DBC_Ctr"={"DBC Path"=path "", "DBC loading channel"=0, "DatabaseId"=0, "DBMessages"=[], "DBSignals"=[]}, "CAN_Config_Array"=[], "CANFD_Config_Array"=[], "CAN_Config_Regs_Array"=[], "CANFD_Config_Regs_Array"=[], "Blf_Log"={"Blf_Log_PATH"=path ""}, "UDS"={"UDS Control"={"UDS Channel Index"=0, "Request ID"=1992, "Response ID"=2015, "Request ID (Func)"=1, "Session Mode"=1, "Reset Mode"=255, "DTC Mask"=0, "GropOfDTC"=0, "Seed Level"=2, "Seed"=[], "Key Level"=0, "Key"=[], "Read Identifier"=0, "UDS Read Data"=[], "ASCII Data"="", "Write Identifier"=0, "UDS Wrtie Data"=[], "IO Control Identifier"=1, "UDS IOControl Data"=[], "IO Control Mode"=0, "UDS IOControl Read Data"=[], "Routine Control Identifier"=0, "UDS RoutineControl Data"=[], "UDS RoutineControl Read Data"=[], "Routine Control Mode"=1, "SupportFDCAN"=TRUE, "time config"={"p2_timeout"=0, "p2_extended"=0, "s3_servertime"=0, "s3_clienttime"=0}, "ServiceLayer"={"FilledByte"=0, "STMin"=10, "BlockSize"=10, "FCDelay"=10, "MaxLength"=4095}, "Request"=[], "Respond"=[]}, "DiagModuleIndex"=1984}}, "CAN_Buffer"=[], "CANFD_Buffer"=[], "error in"={"status"=FALSE, "code"=0, "source"=""}, "CAN_Period_Datas"=[], "CANFD_period_Datas"=[], "CAN_Filtering_Datas"=[], "CANFD_Filtering_Datas"=[], "AsynCall?"=FALSE} ("Data"), "Data.Config_parameter.Bus_Type"="Bus_Type", "Data.Config_parameter.Channels used"="Channels used", "Data.Config_parameter.DLL_PATH"="DLL_PATH", "Data.Config_parameter.Channel"="Channel", "Data.Config_parameter.Read message type"="Read message type", "Data.Blf_Log.Blf_Log_PATH"="BLF_Log_PATH", "Data.Config_parameter.REC_Channel"="REC_Channel") -> (w1309:T10)
            n465 = case shown="0, 默认" "async&sync" {
              tunnel: [T8."Disabled and Grayed Out" ("禁用") T8."Enabled" ("禁用")] -> w1288
              frame 0, Default {
              }
              frame 1 {
              }
            }
            n466 = Bundle By Name(cluster=w1309, "Data.Send_parameter.SendData"="SendData", "Data.Send_parameter.Data Length"="Data Length", "Data.Send_parameter.ID"="ID", "Data.Send_parameter.Frame Format"="Frame Format", "Data.Send_parameter.Frame Type"="Frame Type", "Data.Send_parameter.BRS"="BRS", "Data.Send_parameter.FD Frame"="FD Frame", "Data.Send_parameter.async&sync"="async&sync", "Data.Send_parameter.Timeout"="Timeout") -> (w1303:T10)
            n467 = property on="Timeout" class="DigNum (严格)"("DisabledEnum"=w1288) -> ()  [unwired: 2 in, 2 out]
            n468 = case shown="0, 默认" "Bus_Type" {
              tunnel: [T8."Disabled and Grayed Out" ("禁用") T8."Enabled" ("禁用")] -> w1284
              tunnel: [T8."Enabled" ("禁用") T8."Disabled and Grayed Out" ("禁用")] -> w1283
              frame 0, Default {
              }
              frame 1 {
              }
            }
            n469 = Bundle By Name(cluster=w1303, "Data.DBC_Ctr.DBC Path"="DBC Path", "Data.DBC_Ctr.DBC loading channel"="DBC loading channel") -> (w1294:T10)
            n470 = Bundle By Name(cluster=w1294, "Data.CAN_Config_Array"="CAN_Config_Array", "Data.CANFD_Config_Array"="CANFD_Config_Array", "Data.CAN_Config_Regs_Array"="CAN_Config_Regs_Array", "Data.CANFD_Config_Regs_Array"="CANFD_Config_Regs_Array") -> (w1295:T10)
            n471 = property on="FD Frame" class="Ring (严格)"("DisabledEnum"=w1284) -> ()  [unwired: 2 in, 2 out]
            n472 = property on="BRS" class="Enum (严格)"("DisabledEnum"=w1284) -> ()  [unwired: 2 in, 2 out]
            n473 = property on="CANFD_Config_Array" class="Arr (严格)"("DisabledEnum"=w1284) -> ()  [unwired: 2 in, 2 out]
            n474 = property on="CAN_Config_Array" class="Arr (严格)"("DisabledEnum"=w1283) -> ()  [unwired: 2 in, 2 out]
            n475 = property on="CAN_Config_Regs_Array" class="Arr (严格)"("DisabledEnum"=w1283) -> ()  [unwired: 2 in, 2 out]
            n476 = property on="CANFD_Config_Regs_Array" class="Arr (严格)"("DisabledEnum"=w1284) -> ()  [unwired: 2 in, 2 out]
            n477 = To Variant(anything=w1295) -> (Variant=w1308:variant)
            n478 = Bundle By Name(cluster=T20 {"Sender"="", "receiver"="", "message"="", "data"=variant} ("Communication message"), "message"="Config update", "data"=w1308) -> (w1310:T20)
          }
          event "Diagram shown": Value Change {
            n479 = event-data() -> ("NewVal"=w1320:bool)  [unwired: 1 in, 5 out]
            n480 = To Variant(anything=w1320) -> (Variant=w1321:variant)
            n481 = Bundle By Name(cluster=T20 {"Sender"="", "receiver"="", "message"="", "data"=variant} ("Communication message"), "message"="Diagram shown", "data"=w1321) -> (w1322:T20)
          }
          event "Config": Value Change {
            n482 = event-data() -> ()  [unwired: 1 in, 6 out]
            n483 = Bundle By Name(cluster=T20 {"Sender"="", "receiver"="", "message"="", "data"=variant} ("Communication message"), "message"="Init") -> (w1329:T20)
          }
          event "Sampling point": Value Change {
            n484 = event-data() -> ("NewVal"=w1333:bool)  [unwired: 1 in, 5 out]
            n485 = case shown="假" w1333 {
              tunnel: [enum32{"Ordinary", "Advanced"}."Ordinary" ("Advance_Tag") enum32{"Ordinary", "Advanced"}."Advanced" ("Advance_Tag")] -> w1334
              frame False {
              }
              frame True {
              }
            }
            n486 = local write "Advance_Tag"(w1334) -> ()
          }
          event "Connect": Value Change {
            n487 = event-data() -> ()  [unwired: 1 in, 6 out]
            n488 = Bundle By Name(cluster=T20 {"Sender"="", "receiver"="", "message"="", "data"=variant} ("Communication message"), "message"="Connect") -> (w1339:T20)
          }
          event "Disconnect": Value Change {
            n489 = event-data() -> ()  [unwired: 1 in, 6 out]
            n490 = Bundle By Name(cluster=T20 {"Sender"="", "receiver"="", "message"="", "data"=variant} ("Communication message"), "message"="Disconnect") -> (w1344:T20)
          }
          event "TS_Mapping": Value Change {
            n491 = event-data() -> ("NewVal"=w1348:bool)  [unwired: 1 in, 5 out]
            n492 = case shown="真" w1348 {
              tunnel: [T8."Disabled and Grayed Out" ("禁用") T8."Enabled" ("禁用")] -> w1349
              frame False {
                n493 = local write "CH_Mapping"(FALSE ("CH_Mapping")) -> ()
              }
              frame True {
              }
            }
            n494 = property on="CH_Mapping" class="Bool (严格)"("DisabledEnum"=w1349) -> ()  [unwired: 2 in, 2 out]
          }
          event "DIS_REC": Value Change {
            n495 = event-data() -> ("NewVal"=w1355:bool)  [unwired: 1 in, 5 out]
            n496 = To Variant(anything=w1355) -> (Variant=w1356:variant)
            n497 = Bundle By Name(cluster=T20 {"Sender"="", "receiver"="", "message"="", "data"=variant} ("Communication message"), "message"="DIS_REC", "data"=w1356) -> (w1357:T20)
          }
          event "Export": Value Change {
            n498 = event-data() -> ()  [unwired: 1 in, 6 out]
            n499 = Bundle By Name(cluster=T20 {"Sender"="", "receiver"="", "message"="", "data"=variant} ("Communication message"), "message"="Export") -> (w1363:T20)
          }
          event "Import": Value Change {
            n500 = event-data() -> ()  [unwired: 1 in, 6 out]
            n501 = Bundle By Name(cluster=T20 {"Sender"="", "receiver"="", "message"="", "data"=variant} ("Communication message"), "message"="Import") -> (w1368:T20)
          }
          event "Sending": Value Change {
            n502 = event-data() -> ()  [unwired: 1 in, 6 out]
            n503 = To Variant(anything="Cycle") -> (Variant=w1373:variant)
            n504 = Bundle By Name(cluster=T20 {"Sender"="", "receiver"="", "message"="", "data"=variant} ("Communication message"), "message"="Sending", "data"=w1373) -> (w1375:T20)
          }
          event "Clear": Value Change {
            n505 = event-data() -> ()  [unwired: 1 in, 6 out]
            n506 = Bundle By Name(cluster=T20 {"Sender"="", "receiver"="", "message"="", "data"=variant} ("Communication message"), "message"="Clear") -> (w1380:T20)
          }
          event "Periodic_Send": Value Change {
            n507 = event-data() -> ()  [unwired: 1 in, 6 out]
            n508 = Bundle By Name(cluster=T20 {"Sender"="", "receiver"="", "message"="", "data"=variant} ("Communication message"), "message"="Periodic_Send") -> (w1385:T20)
          }
          event "Filtering": Value Change {
            n509 = event-data() -> ()  [unwired: 1 in, 6 out]
            n510 = Bundle By Name(cluster=T20 {"Sender"="", "receiver"="", "message"="", "data"=variant} ("Communication message"), "message"="Filtering") -> (w1390:T20)
          }
          event "DBC_Send": Value Change {
            n511 = event-data() -> ()  [unwired: 1 in, 6 out]
            n512 = Bundle By Name(cluster=T20 {"Sender"="", "receiver"="", "message"="", "data"=variant} ("Communication message"), "message"="DBC_Send") -> (w1394:T20)
          }
          event "UDS": Value Change {
            n513 = event-data() -> ()  [unwired: 1 in, 6 out]
            n514 = Bundle By Name(cluster=T20 {"Sender"="", "receiver"="", "message"="", "data"=variant} ("Communication message"), "message"="UDS") -> (w1399:T20)
          }
          event "Load_DBC": Value Change {
            n515 = event-data() -> ()  [unwired: 1 in, 6 out]
            n516 = Bundle By Name(cluster=T20 {"Sender"="", "receiver"="", "message"="", "data"=variant} ("Communication message"), "message"="Load_DBC") -> (w1405:T20)
          }
          event "Unload_DBC": Value Change {
            n517 = event-data() -> ()  [unwired: 1 in, 6 out]
            n518 = Bundle By Name(cluster=T20 {"Sender"="", "receiver"="", "message"="", "data"=variant} ("Communication message"), "message"="Unload_DBC") -> (w1410:T20)
          }
          event "Tree control": Mouse Up {
            n519 = event-data() -> ("CtlRef"=w1415:refnum<vi>)  [unwired: 1 in, 7 out]
            n520 = To Variant(anything=w1415) -> (Variant=w1414:variant)
            n521 = Bundle By Name(cluster=T20 {"Sender"="", "receiver"="", "message"="", "data"=variant} ("Communication message"), "message"="DBC_Define", "data"=w1414) -> (w1416:T20)
          }
          event "Start Log": Value Change {
            n522 = event-data() -> ()  [unwired: 1 in, 6 out]
            n523 = Bundle By Name(cluster=T20 {"Sender"="", "receiver"="", "message"="", "data"=variant} ("Communication message"), "message"="Start Log") -> (w1422:T20)
          }
          event "Stop Log": Value Change {
            n524 = event-data() -> ()  [unwired: 1 in, 6 out]
            n525 = Bundle By Name(cluster=T20 {"Sender"="", "receiver"="", "message"="", "data"=variant} ("Communication message"), "message"="Stop Log") -> (w1427:T20)
          }
          event "GetCount_DBC": Value Change {
            n526 = event-data() -> ()  [unwired: 1 in, 6 out]
            n527 = Bundle By Name(cluster=T20 {"Sender"="", "receiver"="", "message"="", "data"=variant} ("Communication message"), "message"="GetCount_DBC") -> (w1432:T20)
          }
          event User Event {
            n528 = event-data() -> ("Quit"=w1439:string)  [unwired: 1 in]
            n529 = Equal?(x=w1439, y="Quit") -> (x = y?=w1437:bool)
          }
          event Panel Close? {
            w1445 = TRUE ("放弃？")
            n530 = event-data() -> ()  [unwired: 1 in, 4 out]
            n531 = Enqueue Element(queue=w1444, element=T20 {"Sender"="", "receiver"="", "message"="Quit", "data"=variant} ("Communication message")) -> (queue out=w1442:refnum<queue>)  [unwired: 2 in, 2 out]
            n532 = event-data("Discard?"=w1445) -> ()  [unwired: 1 in, 1 out]
          }
          event "STOP": Value Change {
            n533 = event-data() -> ()  [unwired: 1 in, 6 out]
            n534 = Enqueue Element(queue=w1449, element=T20 {"Sender"="", "receiver"="", "message"="Quit", "data"=variant} ("Communication message")) -> (queue out=w1447:refnum<queue>)  [unwired: 2 in, 2 out]
          }
        }
        n535 = Unbundle By Name(w1262) -> ("message"=w1261:string)
        n536 = case shown="\"default\", 默认" w1261 {
          tunnel: w1265 -> [w1272 w1274]
          tunnel: w1263 -> [w1271 w1273]
          tunnel: w1262 -> [w1270 _]
          tunnel: [w1269 w1274] -> _
          tunnel: [w1268 w1273] -> _
          frame "default", Default {
            n537 = Enqueue Element(queue=w1272, element=w1270, error in (no error)=w1271) -> (queue out=w1269:refnum<queue>, error out=w1268:errorcluster)  [unwired: 1 in, 1 out]
          }
          frame "" {
          }
        }
      }
      n538 = Release Queue(queue=w87, error in (no error)=w86) -> ()  [unwired: 1 in, 3 out]
    }
  }
  n539 = Release Queue(queue=w11, error in (no error)=w10) -> (error out=w9:errorcluster)  [unwired: 1 in, 2 out]
  n540 = Destroy User Event(user event=w1) -> (error out=w3:errorcluster)  [unwired: 1 in]
  n541 = property class="App"(error in=w9) -> (error out=w8:errorcluster, "App.Kind"=w7:T30)  [unwired: 1 in, 1 out]
  n542 = Unregister For Events(event registration refnum=w2, error in=w3) -> ()  [unwired: 1 out]
  n543 = case shown="\"Run Time System\"" w7 {
    tunnel: w8 -> [_ _ w1451 _ _ _ _]
    frame "invalid app kind", Default {
    }
    frame "Development System" {
    }
    frame "Run Time System" {
      n544 = invoke class="VI" method="FP.Close"(error in=w1451) -> ()  [unwired: 2 in, 3 out]
    }
    frame "Student Edition" {
    }
    frame "Embedded LabVIEW" {
    }
    frame "Evaluation" {
    }
    frame "Custom" {
    }
  }
